vi "BRig_RT_panel_Laser1_v1,10.vi"(7 "input_setValues":bool, 9 "input_dataExp":u16[](array[numeric]), 11 "input_dataLC":u16[](array[numeric])) -> (1 "output_dataExp":u16[](array[numeric]), 3 "output_dataLC":u16[](array[numeric]))   [LabVIEW 2014]
panel:
  in  "Numeric 2":dbl
  in  "Numeric":dbl
  in  "LC_Cue2_PostR_Count":u16
  in  "LC_Cue2_PostR_delayOpt":bool
  in  "LC_Cue2_PostR_Probability":u16
  in  "LC_Cue2_PostR_Block":u16(slide) max=2 step=1 scale=0.0..2.0
  in  "LC_Cue2_PostR_OnOff":bool
  in  "LC_Cue2_PostR_Tdelay":u16
  in  "LC_ENL2_PostR_delayOpt":bool
  in  "LC_ENL2_PostR_Count":u16
  in  "LC_ENL2_PostR_Probability":u16 max=100 step=1
  in  "LC_ENL2_PostR_Block":u16(slide) max=2 step=1 scale=0.0..2.0
  in  "LC_ENL2_PostR_OnOff":bool
  in  "LC_ENL2_PostR_Tdelay":u16
  in  "LC_Cue2_PreR_Count":u16
  in  "LC_Cue2_First_Count":u16
  in  "LC_Cue2_PreR_delayOpt":bool
  in  "LC_ENL2_PreR_delayOpt":bool
  in  "LC_ENL2_PreR_Count":u16
  in  "LC_ENL2_First_Count":u16
  in  "LC_Cue2_First_delayOpt":bool
  in  "LC_ENL2_First_delayOpt":bool
  in  "LC_Cue2_PreR_Probability":u16
  in  "LC_Cue2_PreR_Block":u16(slide) max=2 step=1 scale=0.0..2.0
  in  "LC_Cue2_PreR_OnOff":bool
  in  "LC_Cue2_First_Probability":u16
  in  "LC_Cue2_First_Block":u16(slide) max=2 step=1 scale=0.0..2.0
  in  "LC_Cue2_First_OnOff":bool
  in  "LC_ENL2_PreR_Probability":u16 max=100 step=1
  in  "LC_ENL2_PreR_Block":u16(slide) max=2 step=1 scale=0.0..2.0
  in  "LC_ENL2_PreR_OnOff":bool
  in  "LC_ENL2_First_Probability":u16 max=100 step=1
  in  "LC_ENL2_First_Block":u16(slide) max=2 step=1 scale=0.0..2.0
  in  "LC_Cue2_PreR_Tdelay":u16
  in  "LC_ENL2_PreR_Tdelay":u16
  in  "LC_Cue2_First_Tdelay":u16
  in  "LC_ENL2_First_Tdelay":u16
  in  "LC_ENL2_First_OnOff":bool
  out "LaserPulseTrain":cluster{u16[], u16[]}(graph)
  in  "LED_baseline":bool
  in  "Laser_power_step":dbl
  in  "Laser_power_max":dbl
  in  "Laser_power_min":dbl
  in  "Laser_Tshutter":u16=2
  in  "Laser_Freq":u16=10
  in  "Laser_Tpeak":u16=2
  in  "Laser_T":u16
  in  "LC_Sel_PostR_Count":u16
  in  "LC_Sel_PostR_Probability":u16
  in  "LC_Sel_PostR_Block":u16(slide) max=2 step=1 scale=0.0..2.0
  in  "LC_Sel_PostR_OnOff":bool
  in  "LC_Sel_PostR_Tdelay":u16
  in  "LC_Cue_PostR_Count":u16
  in  "LC_Cue_PostR_delayOpt":bool
  in  "LC_Cue_PostR_Probability":u16
  in  "LC_Cue_PostR_Block":u16(slide) max=2 step=1 scale=0.0..2.0
  in  "LC_Cue_PostR_OnOff":bool
  in  "LC_Cue_PostR_Tdelay":u16
  in  "LC_ENL_PostR_delayOpt":bool
  in  "LC_ENL_PostR_Count":u16
  in  "LC_ENL_PostR_Probability":u16 max=100 step=1
  in  "LC_ENL_PostR_Block":u16(slide) max=2 step=1 scale=0.0..2.0
  in  "LC_ENL_PostR_OnOff":bool
  in  "LC_ENL_PostR_Tdelay":u16
  in  "LC_Sel_PreR_Count":u16
  in  "LC_Sel_First_Count":u16
  in  "LC_Sel_PreR_Probability":u16
  in  "LC_Sel_PreR_Block":u16(slide) max=2 step=1 scale=0.0..2.0
  in  "LC_Sel_PreR_OnOff":bool
  in  "LC_Sel_First_Probability":u16
  in  "LC_Sel_First_Block":u16(slide) max=2 step=1 scale=0.0..2.0
  in  "LC_Sel_First_OnOff":bool
  in  "LC_Sel_PreR_Tdelay":u16
  in  "LC_Sel_First_Tdelay":u16
  in  "LC_Cue_PreR_Count":u16
  in  "LC_Cue_First_Count":u16
  in  "LC_Cue_PreR_delayOpt":bool
  in  "LC_ENL_PreR_delayOpt":bool
  in  "LC_ENL_PreR_Count":u16
  in  "LC_ENL_First_Count":u16
  in  "LC_Cue_First_delayOpt":bool
  in  "LC_ENL_First_delayOpt":bool
  in  "LC_Wrong_Probability":u16
  in  "LC_Wrong_Trial":u16(slide) max=2 step=1 scale=0.0..2.0
  in  "LC_Wrong_Block":u16(slide) max=2 step=1 scale=0.0..2.0
  in  "LC_Wrong_OnOff":bool
  in  "LC_Reward_Probability":u16
  in  "LC_Reward_Trial":u16(slide) max=2 step=1 scale=0.0..2.0
  in  "LC_Reward_Block":u16(slide) max=2 step=1 scale=0.0..2.0
  in  "LC_Reward_OnOff":bool
  in  "LC_Cue_PreR_Probability":u16
  in  "LC_Cue_PreR_Block":u16(slide) max=2 step=1 scale=0.0..2.0
  in  "LC_Cue_PreR_OnOff":bool
  in  "LC_Cue_First_Probability":u16
  in  "LC_Cue_First_Block":u16(slide) max=2 step=1 scale=0.0..2.0
  in  "LC_Cue_First_OnOff":bool
  in  "LC_ENL_PreR_Probability":u16 max=100 step=1
  in  "LC_ENL_PreR_Block":u16(slide) max=2 step=1 scale=0.0..2.0
  in  "LC_ENL_PreR_OnOff":bool
  in  "LC_ENL_First_Probability":u16 max=100 step=1
  in  "LC_ENL_First_Block":u16(slide) max=2 step=1 scale=0.0..2.0
  in  "LC_Wrong_Tdelay":u16
  in  "LC_Cue_PreR_Tdelay":u16
  in  "LC_ENL_PreR_Tdelay":u16
  in  "LC_Reward_Tdelay":u16
  in  "LC_Cue_First_Tdelay":u16
  in  "LC_ENL_First_Tdelay":u16
  in  "LC_ENL_First_OnOff":bool
  # "Laser1 Control\n                               On/Off      Block        Probability [%]   Delay [ms]                              Count"
  # "On/Off      Block        Probability [%]   Delay [ms]                              Count"
  # "Enforced\nNonLick"
  # "Enforced\nNonLick\n     2"
  # "from end"
  # "from end"
  # "First\nTrial"
  # "First\nTrial"
  # "from start"
  # "from start"
  # "from end"
  # "from end"
  # "PreReward\nTrials"
  # "PreReward\nTrials"
  # "from start"
  # "from start"
  # "from end"
  # "from end"
  # "PostReward\nTrials"
  # "PostReward\nTrials"
  # "from start"
  # "from start"
  # "Cue"
  # "Cue\n  2"
  # "from end"
  # "from end"
  # "First\nTrial"
  # "First\nTrial"
  # "from start"
  # "from start"
  # "from end"
  # "from end"
  # "PreReward\nTrials"
  # "PreReward\nTrials"
  # "from start"
  # "from start"
  # "from end"
  # "from end"
  # "PostReward\nTrials"
  # "PostReward\nTrials"
  # "from start"
  # "from start"
  # "Selection"
  # "from start"
  # "First\nTrial"
  # "from start"
  # "PreReward\nTrials"
  # "from start"
  # "PostReward\nTrials"
  # "Laser1 Parameters"
  # "Laser1 Response\n           On/Off      Block           Trial     Probability %  Delay [ms]"
  # "Frequency\n[Hz]"
  # "Selection\nReward"
  # "Timing [ms]\n Duration     Peak Width   Shutter"
  # "Selection\nWrong"
  # "Laser Power [V]\nMin          Max              Step"
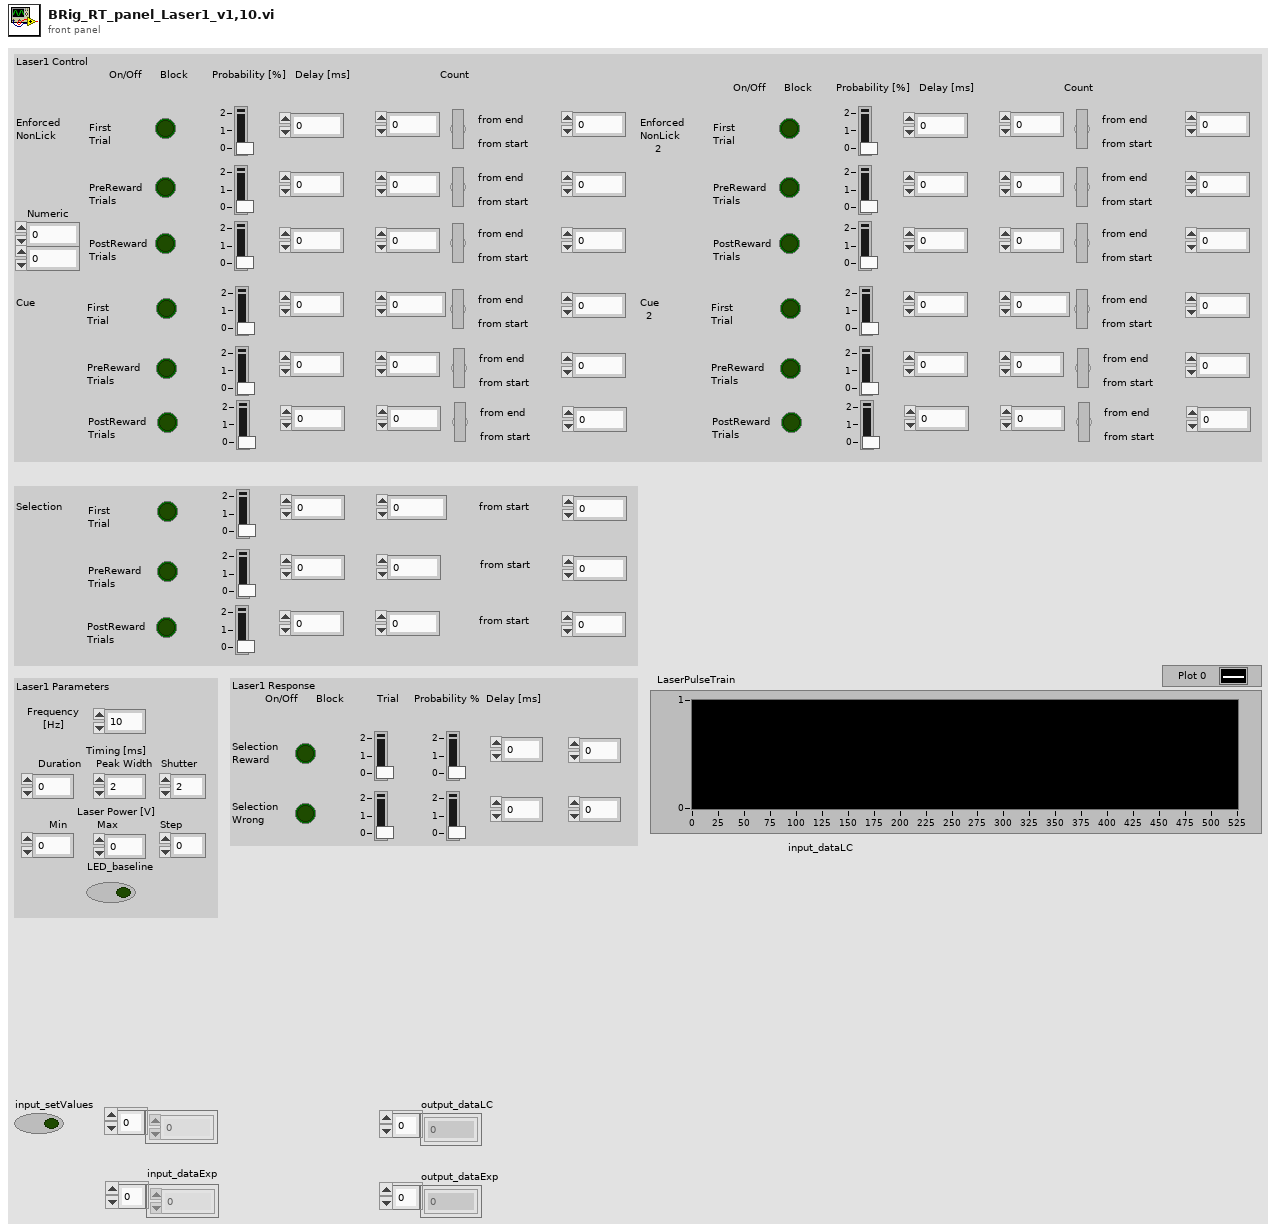
[diagram p1: front panel]
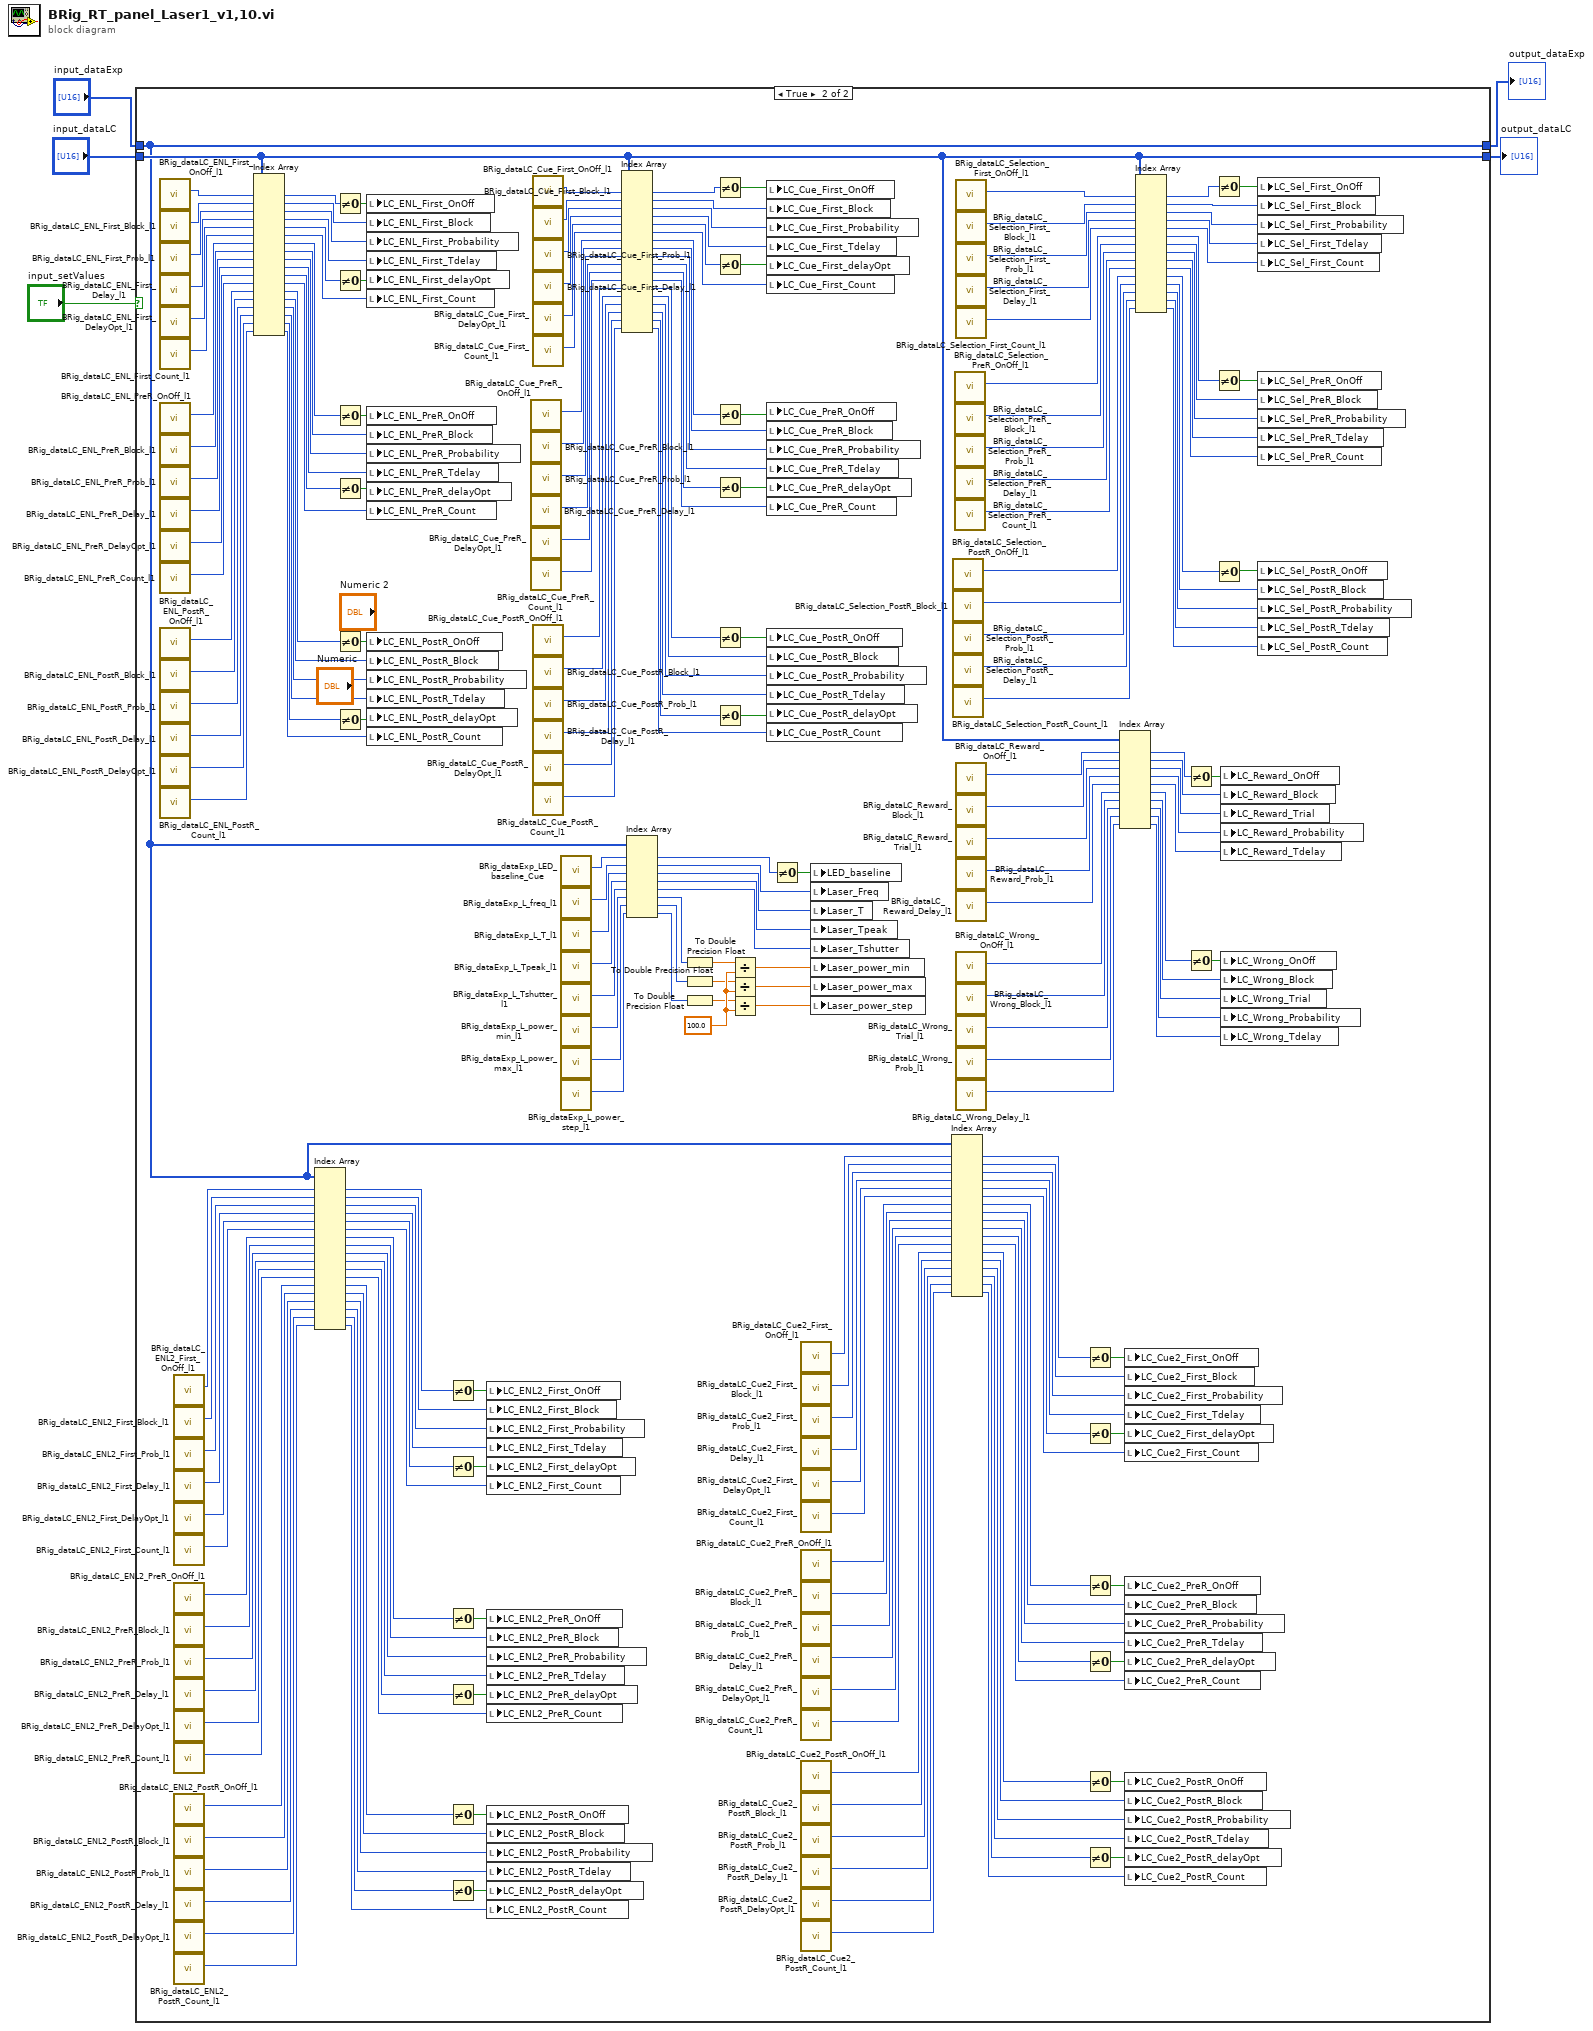
[diagram p0: block diagram]
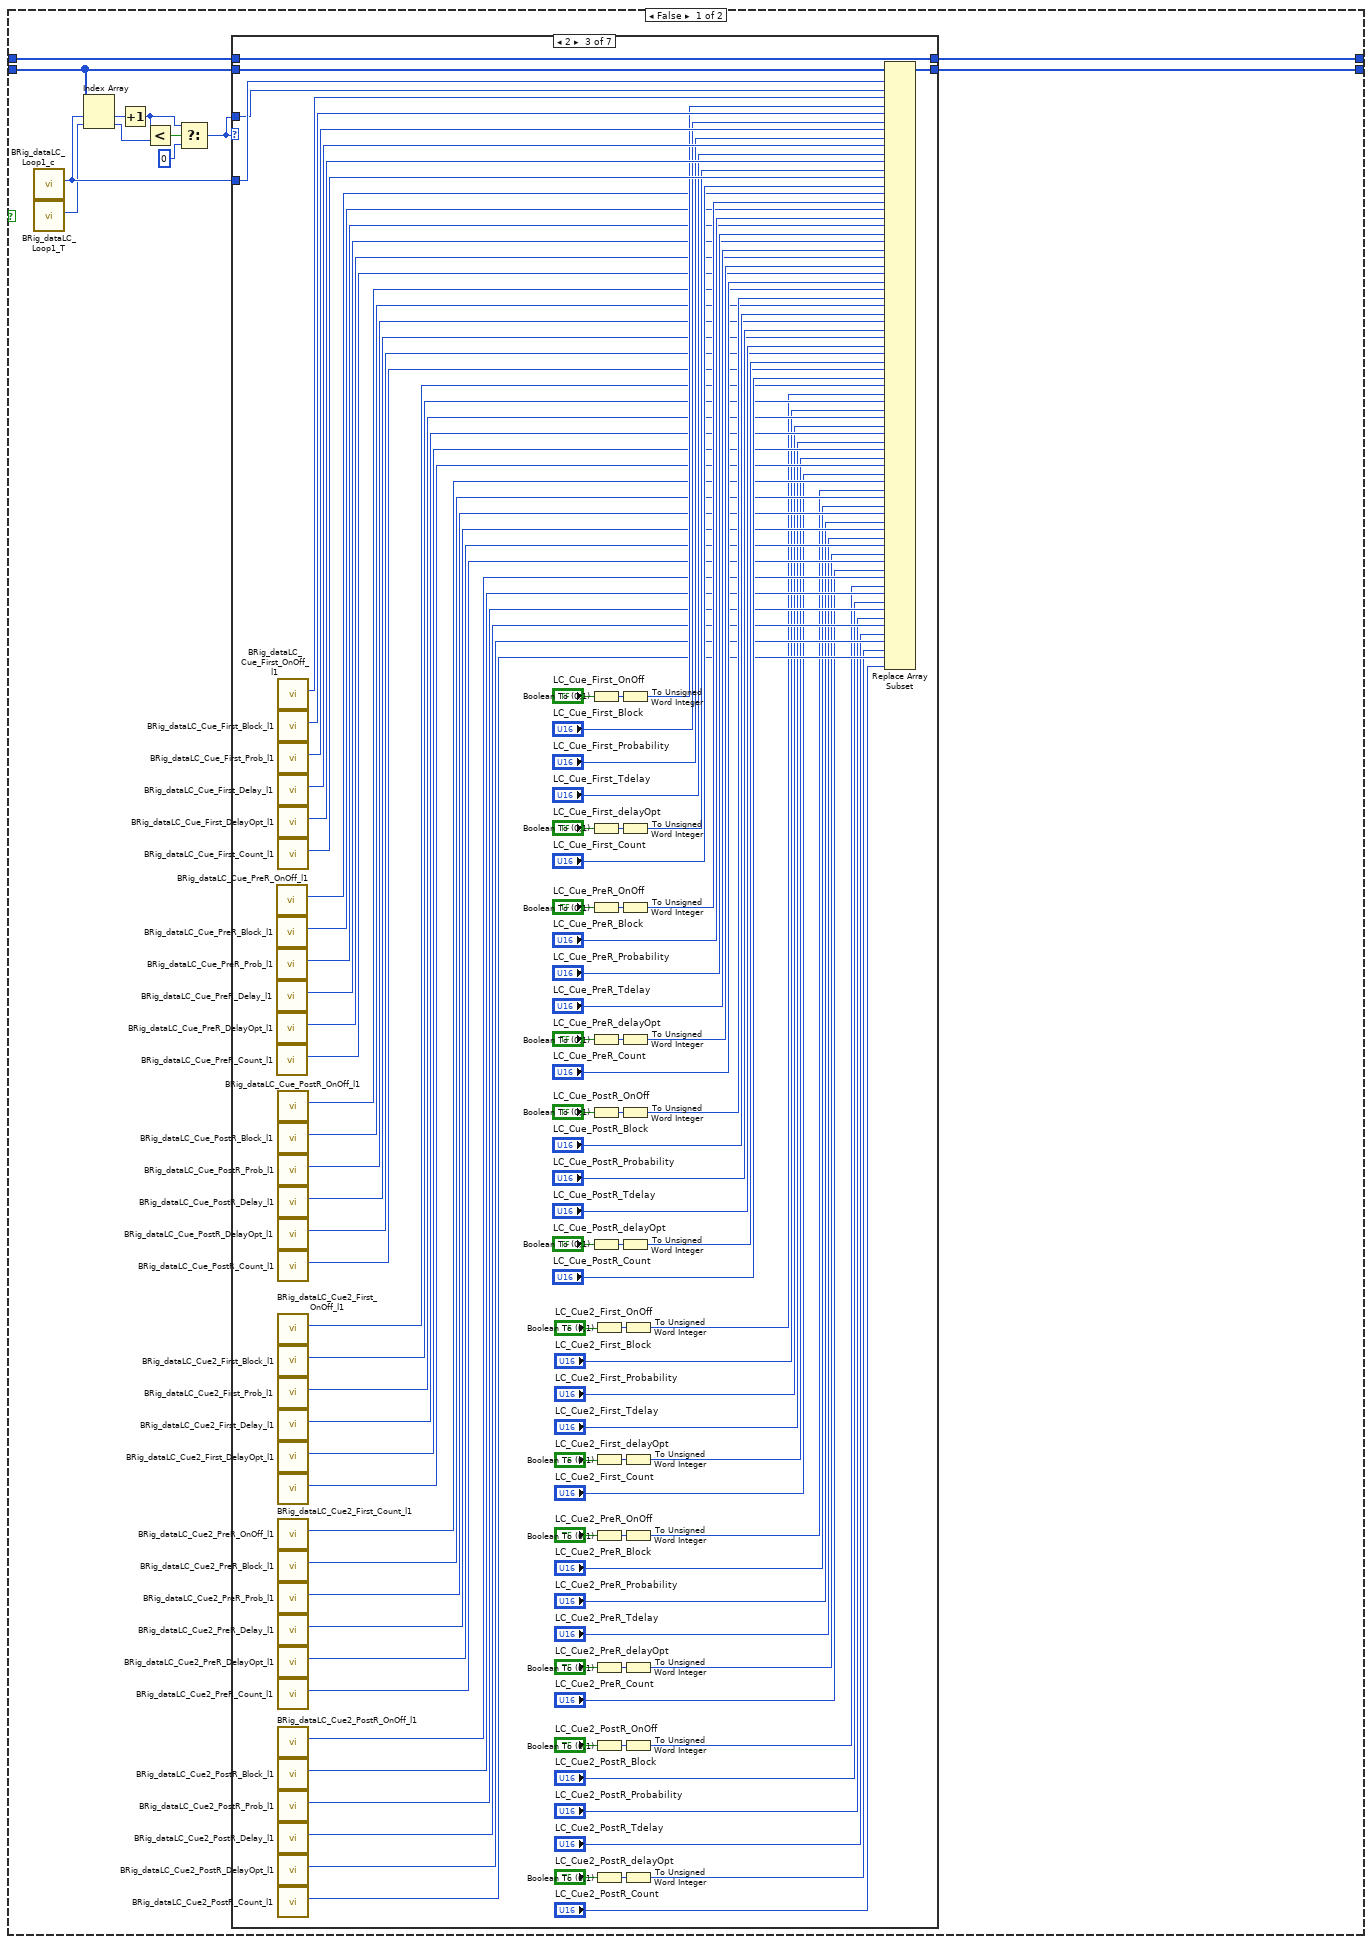
[diagram p2: hidden frame]
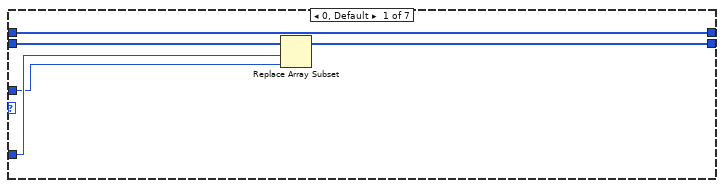
[diagram p3: hidden frame]
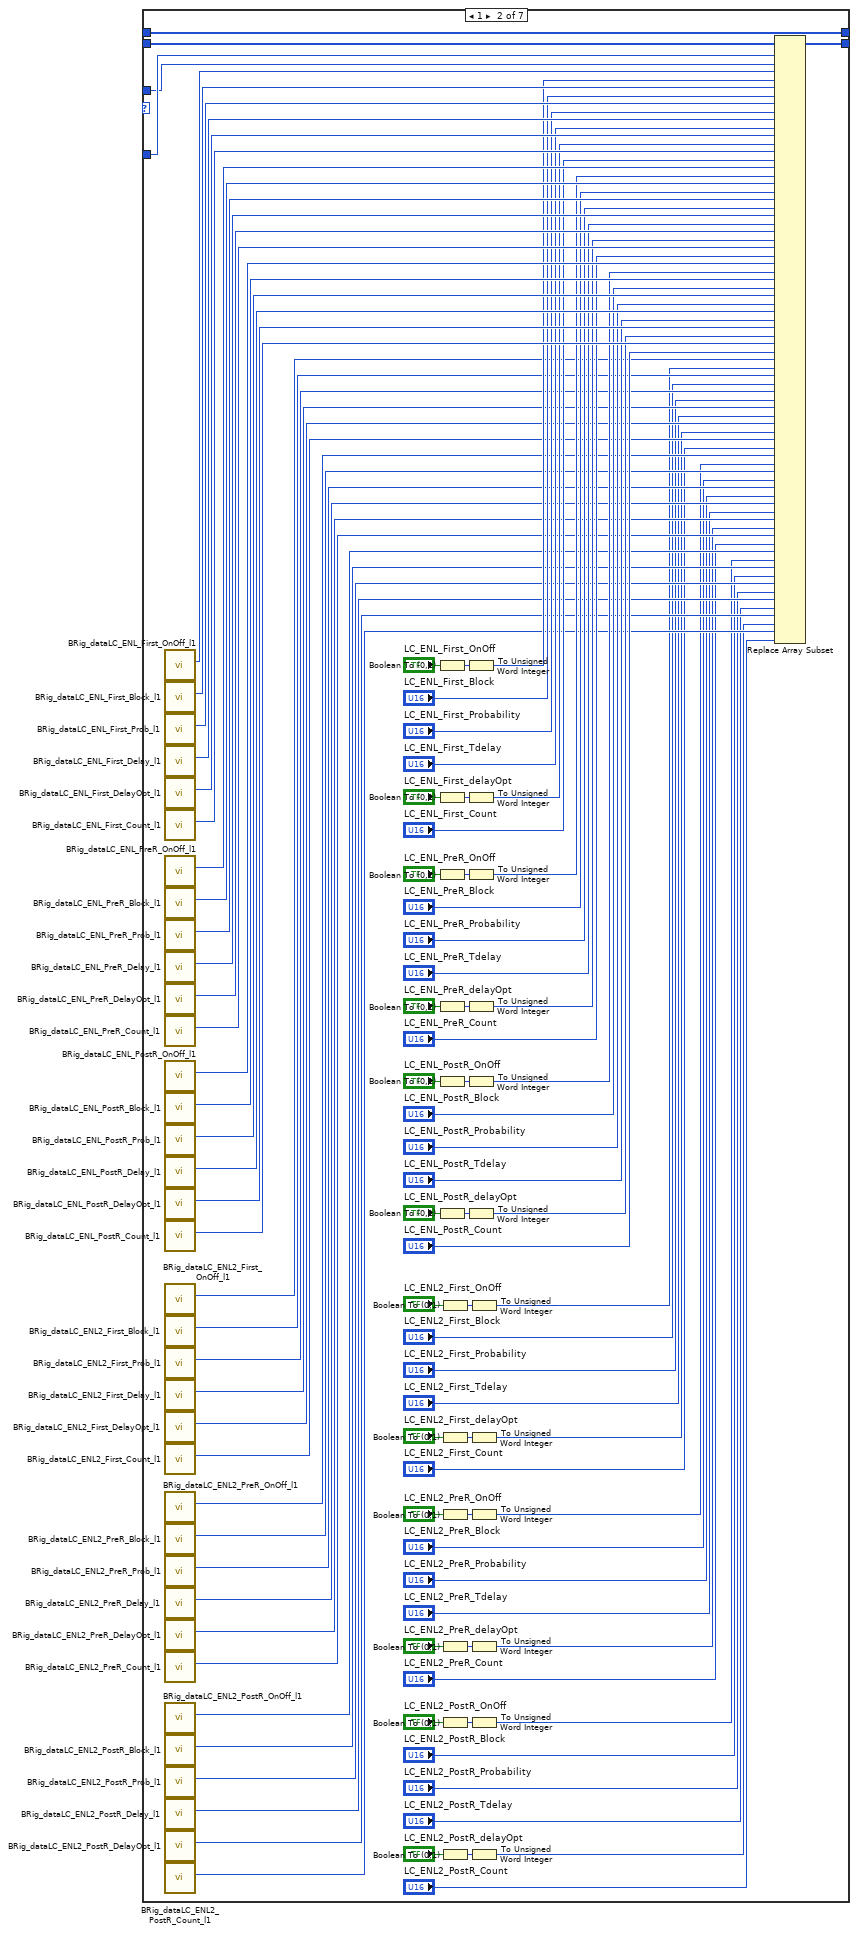
[diagram p4: hidden frame]
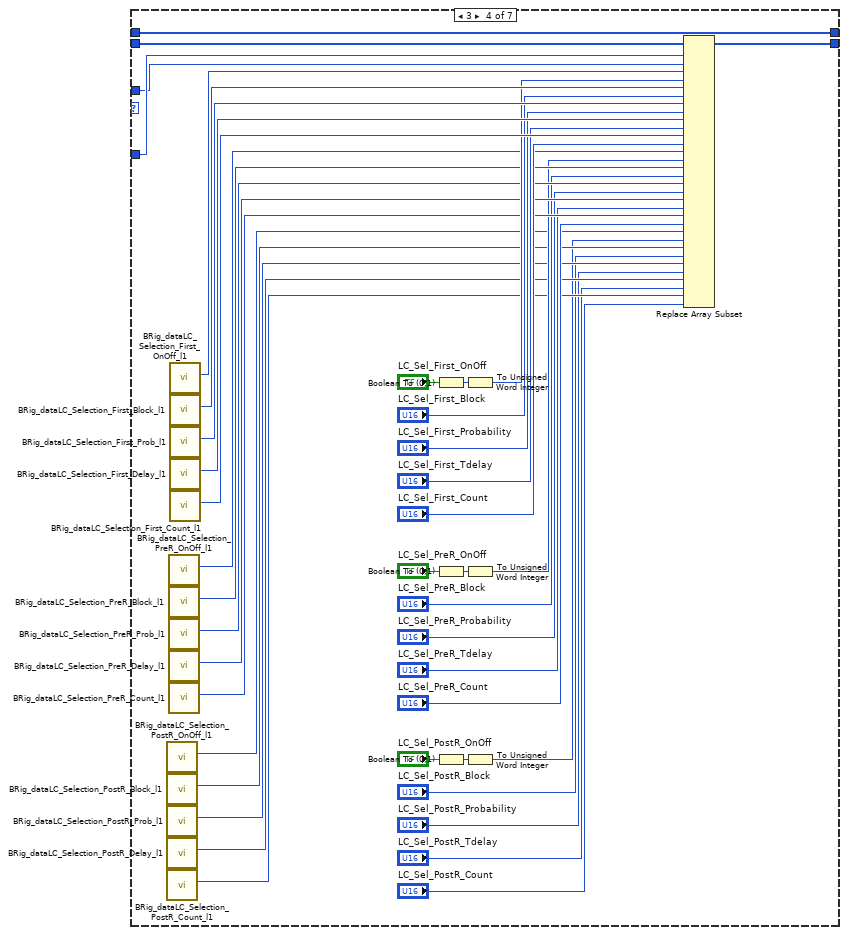
[diagram p5: hidden frame]
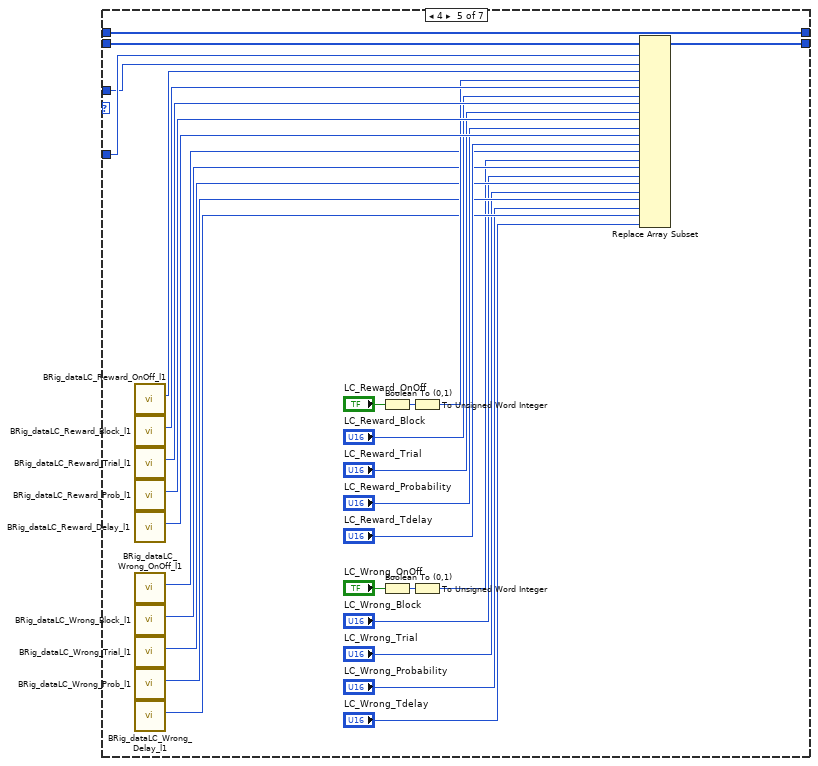
[diagram p6: hidden frame]
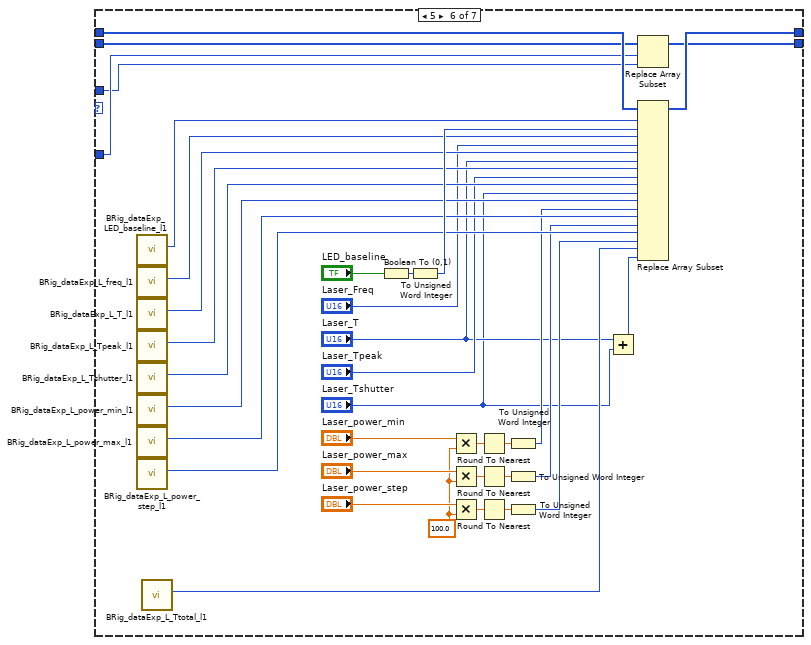
[diagram p7: hidden frame]
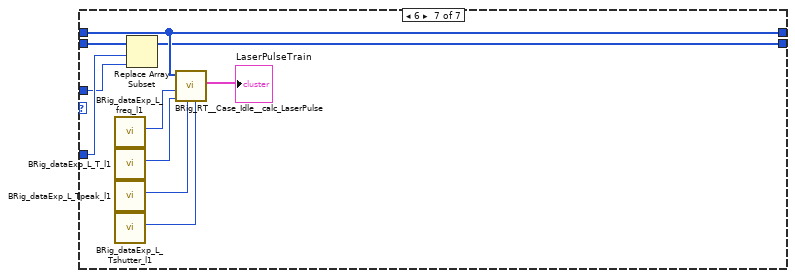
[diagram p8: hidden frame]
diagram:
  n1 = case shown="True" "input_setValues" {
    tunnel: "input_dataLC" -> [w17 w462]
    tunnel: [w11 w462] -> w4
    tunnel: "input_dataExp" -> [w7 w377]
    tunnel: [w6 w377] -> w1
    frame False {
      n2 = call "BRig_dataLC_Loop1_c.vi"() -> ("output_Loop1_c"=w10:i32)  [unwired: 11 in]
      n3 = call "BRig_dataLC_Loop1_T.vi"() -> ("output_Loop1_T"=w9:i32)  [unwired: 11 in]
      n4 = Index Array(array=w17, index #1=w10, index #2=w9) -> (element #1=w16:u16, element #2=w15:u16)
      n5 = Increment(x=w16) -> (x+1=w12:u16)
      n6 = Less?(x=w12, y=w15) -> (x < y?=w14:bool)
      n7 = Select(t=w12, s=w14, f=u16 0) -> (s? t:f=w8:u16)
      n8 = case shown="2" w8 {
        tunnel: w17 -> [w22 w123 w224 w265 w294 w299 w338]
        tunnel: w10 -> [w20 w73 w186 w227 w268 w297 w336]
        tunnel: w8 -> [w19 w72 w185 w226 w267 w296 w335]
        tunnel: [w21 w116 w223 w264 w293 w298 w337] -> w11
        tunnel: w7 -> [w18 w71 w172 w225 w266 w301 w340]
        tunnel: [w18 w71 w172 w225 w266 w300 w340] -> w6
        frame 0, Default {
          n9 = Replace Array Subset(array=w22, new element=w19, index=w20) -> (w21:u16[])
        }
        frame 1 {
          n10 = call "BRig_dataLC_ENL_First_OnOff_l1.vi"() -> ("output_ENL_First_OnOff"=w122:i32)  [unwired: 11 in]
          n11 = call "BRig_dataLC_ENL_First_Block_l1.vi"() -> ("output_ENL_First_Block"=w121:i32)  [unwired: 11 in]
          n12 = call "BRig_dataLC_ENL_First_Prob_l1.vi"() -> ("output_ENL_First_Prob"=w120:i32)  [unwired: 11 in]
          n13 = call "BRig_dataLC_ENL_First_Delay_l1.vi"() -> ("output_ENL_First_Delay"=w119:i32)  [unwired: 11 in]
          n14 = call "BRig_dataLC_ENL_First_DelayOpt_l1.vi"() -> ("output_ENL_First_DelayOpt"=w118:i32)  [unwired: 11 in]
          n15 = call "BRig_dataLC_ENL_First_Count_l1.vi"() -> ("output_ENL_First_Count"=w117:i32)  [unwired: 11 in]
          n16 = call "BRig_dataLC_ENL_PreR_OnOff_l1.vi"() -> ("output_ENL_PreR_OnOff"=w115:i32)  [unwired: 11 in]
          n17 = call "BRig_dataLC_ENL_PreR_Block_l1.vi"() -> ("output_ENL_PreR_Block"=w114:i32)  [unwired: 11 in]
          n18 = call "BRig_dataLC_ENL_PreR_Prob_l1.vi"() -> ("output_ENL_PreR_Prob"=w113:i32)  [unwired: 11 in]
          n19 = call "BRig_dataLC_ENL_PreR_Delay_l1.vi"() -> ("output_ENL_PreR_Delay"=w112:i32)  [unwired: 11 in]
          n20 = call "BRig_dataLC_ENL_PreR_DelayOpt_l1.vi"() -> ("output_ENL_PreR_DelayOpt"=w111:i32)  [unwired: 11 in]
          n21 = call "BRig_dataLC_ENL_PreR_Count_l1.vi"() -> ("output_ENL_PreR_Count"=w110:i32)  [unwired: 11 in]
          n22 = call "BRig_dataLC_ENL_PostR_OnOff_l1.vi"() -> ("output_ENL_PostR_OnOff"=w109:i32)  [unwired: 11 in]
          n23 = call "BRig_dataLC_ENL_PostR_Block_l1.vi"() -> ("output_ENL_PostR_Block"=w108:i32)  [unwired: 11 in]
          n24 = call "BRig_dataLC_ENL_PostR_Prob_l1.vi"() -> ("output_ENL_PostR_Prob"=w107:i32)  [unwired: 11 in]
          n25 = call "BRig_dataLC_ENL_PostR_Delay_l1.vi"() -> ("output_ENL_PostR_Delay"=w106:i32)  [unwired: 11 in]
          n26 = call "BRig_dataLC_ENL_PostR_DelayOpt_l1.vi"() -> ("output_ENL_PostR_DelayOpt"=w105:i32)  [unwired: 11 in]
          n27 = call "BRig_dataLC_ENL_PostR_Count_l1.vi"() -> ("output_ENL_PostR_Count"=w104:i32)  [unwired: 11 in]
          n28 = call "BRig_dataLC_ENL2_First_OnOff_l1.vi"() -> ("output_ENL2_First_OnOff"=w70:i32)  [unwired: 11 in]
          n29 = call "BRig_dataLC_ENL2_First_Block_l1.vi"() -> ("output_ENL2_First_Block"=w69:i32)  [unwired: 11 in]
          n30 = call "BRig_dataLC_ENL2_First_Prob_l1.vi"() -> ("output_ENL2_First_Prob"=w68:i32)  [unwired: 11 in]
          n31 = call "BRig_dataLC_ENL2_First_Delay_l1.vi"() -> ("output_ENL2_First_Delay"=w67:i32)  [unwired: 11 in]
          n32 = call "BRig_dataLC_ENL2_First_DelayOpt_l1.vi"() -> ("output_ENL2_First_DelayOpt"=w66:i32)  [unwired: 11 in]
          n33 = call "BRig_dataLC_ENL2_First_Count_l1.vi"() -> ("output_ENL2_First_Count"=w65:i32)  [unwired: 11 in]
          n34 = call "BRig_dataLC_ENL2_PreR_OnOff_l1.vi"() -> ("output_ENL2_PreR_OnOff"=w64:i32)  [unwired: 11 in]
          n35 = call "BRig_dataLC_ENL2_PreR_Block_l1.vi"() -> ("output_ENL2_PreR_Block"=w63:i32)  [unwired: 11 in]
          n36 = call "BRig_dataLC_ENL2_PreR_Prob_l1.vi"() -> ("output_ENL2_PreR_Prob"=w62:i32)  [unwired: 11 in]
          n37 = call "BRig_dataLC_ENL2_PreR_Delay_l1.vi"() -> ("output_ENL2_PreR_Delay"=w61:i32)  [unwired: 11 in]
          n38 = call "BRig_dataLC_ENL2_PreR_DelayOpt_l1.vi"() -> ("output_ENL2_PreR_DelayOpt"=w60:i32)  [unwired: 11 in]
          n39 = call "BRig_dataLC_ENL2_PreR_Count_l1.vi"() -> ("output_ENL2_PreR_Count"=w59:i32)  [unwired: 11 in]
          n40 = call "BRig_dataLC_ENL2_PostR_OnOff_l1.vi"() -> ("output_ENL2_PostR_OnOff"=w58:i32)  [unwired: 11 in]
          n41 = call "BRig_dataLC_ENL2_PostR_Block_l1.vi"() -> ("output_ENL2_PostR_Block"=w57:i32)  [unwired: 11 in]
          n42 = call "BRig_dataLC_ENL2_PostR_Prob_l1.vi"() -> ("output_ENL2_PostR_Prob"=w56:i32)  [unwired: 11 in]
          n43 = call "BRig_dataLC_ENL2_PostR_Delay_l1.vi"() -> ("output_ENL2_PostR_Delay"=w55:i32)  [unwired: 11 in]
          n44 = call "BRig_dataLC_ENL2_PostR_DelayOpt_l1.vi"() -> ("output_ENL2_PostR_DelayOpt"=w54:i32)  [unwired: 11 in]
          n45 = call "BRig_dataLC_ENL2_PostR_Count_l1.vi"() -> ("output_ENL2_PostR_Count"=w53:i32)  [unwired: 11 in]
          n46 = Boolean To (0,1)(Boolean="LC_ENL_First_OnOff") -> (0, 1=w102:i16)
          n47 = Boolean To (0,1)(Boolean="LC_ENL_First_delayOpt") -> (0, 1=w101:i16)
          n48 = Boolean To (0,1)(Boolean="LC_ENL_PreR_OnOff") -> (0, 1=w99:i16)
          n49 = Boolean To (0,1)(Boolean="LC_ENL_PreR_delayOpt") -> (0, 1=w97:i16)
          n50 = Boolean To (0,1)(Boolean="LC_ENL_PostR_OnOff") -> (0, 1=w95:i16)
          n51 = Boolean To (0,1)(Boolean="LC_ENL_PostR_delayOpt") -> (0, 1=w93:i16)
          n52 = Boolean To (0,1)(Boolean="LC_ENL2_First_OnOff") -> (0, 1=w43:i16)
          n53 = Boolean To (0,1)(Boolean="LC_ENL2_First_delayOpt") -> (0, 1=w42:i16)
          n54 = Boolean To (0,1)(Boolean="LC_ENL2_PreR_OnOff") -> (0, 1=w41:i16)
          n55 = Boolean To (0,1)(Boolean="LC_ENL2_PreR_delayOpt") -> (0, 1=w39:i16)
          n56 = Boolean To (0,1)(Boolean="LC_ENL2_PostR_OnOff") -> (0, 1=w31:i16)
          n57 = Boolean To (0,1)(Boolean="LC_ENL2_PostR_delayOpt") -> (0, 1=w29:i16)
          n58 = To Unsigned Word Integer(number=w102) -> (unsigned 16bit integer=w91:u16)
          n59 = To Unsigned Word Integer(number=w101) -> (unsigned 16bit integer=w87:u16)
          n60 = To Unsigned Word Integer(number=w99) -> (unsigned 16bit integer=w85:u16)
          n61 = To Unsigned Word Integer(number=w97) -> (unsigned 16bit integer=w81:u16)
          n62 = To Unsigned Word Integer(number=w95) -> (unsigned 16bit integer=w79:u16)
          n63 = To Unsigned Word Integer(number=w93) -> (unsigned 16bit integer=w75:u16)
          n64 = To Unsigned Word Integer(number=w43) -> (unsigned 16bit integer=w50:u16)
          n65 = To Unsigned Word Integer(number=w42) -> (unsigned 16bit integer=w46:u16)
          n66 = To Unsigned Word Integer(number=w41) -> (unsigned 16bit integer=w44:u16)
          n67 = To Unsigned Word Integer(number=w39) -> (unsigned 16bit integer=w34:u16)
          n68 = To Unsigned Word Integer(number=w31) -> (unsigned 16bit integer=w32:u16)
          n69 = To Unsigned Word Integer(number=w29) -> (unsigned 16bit integer=w24:u16)
          n70 = Replace Array Subset(array=w123, new element #1=w72, index #1=w73, new element #2=w91, index #2=w122, new element #3="LC_ENL_First_Block", index #3=w121, new element #4="LC_ENL_First_Probability", index #4=w120, new element #5="LC_ENL_First_Tdelay", index #5=w119, new element #6=w87, index #6=w118, new element #7="LC_ENL_First_Count", index #7=w117, new element #8=w85, index #8=w115, new element #9="LC_ENL_PreR_Block", index #9=w114, new element #10="LC_ENL_PreR_Probability", index #10=w113, new element #11="LC_ENL_PreR_Tdelay", index #11=w112, new element #12=w81, index #12=w111, new element #13="LC_ENL_PreR_Count", index #13=w110, new element #14=w79, index #14=w109, new element #15="LC_ENL_PostR_Block", index #15=w108, new element #16="LC_ENL_PostR_Probability", index #16=w107, new element #17="LC_ENL_PostR_Tdelay", index #17=w106, new element #18=w75, index #18=w105, new element #19="LC_ENL_PostR_Count", index #19=w104, new element #20=w50, index #20=w70, new element #21="LC_ENL2_First_Block", index #21=w69, new element #22="LC_ENL2_First_Probability", index #22=w68, new element #23="LC_ENL2_First_Tdelay", index #23=w67, new element #24=w46, index #24=w66, new element #25="LC_ENL2_First_Count", index #25=w65, new element #26=w44, index #26=w64, new element #27="LC_ENL2_PreR_Block", index #27=w63, new element #28="LC_ENL2_PreR_Probability", index #28=w62, new element #29="LC_ENL2_PreR_Tdelay", index #29=w61, new element #30=w34, index #30=w60, new element #31="LC_ENL2_PreR_Count", index #31=w59, new element #32=w32, index #32=w58, new element #33="LC_ENL2_PostR_Block", index #33=w57, new element #34="LC_ENL2_PostR_Probability", index #34=w56, new element #35="LC_ENL2_PostR_Tdelay", index #35=w55, new element #36=w24, index #36=w54, new element #37="LC_ENL2_PostR_Count", index #37=w53) -> (w116:u16[])
        }
        frame 2 {
          n71 = call "BRig_dataLC_Cue_PreR_OnOff_l1.vi"() -> ("output_Cue_PreR_OnOff"=w182:i32)  [unwired: 11 in]
          n72 = call "BRig_dataLC_Cue_PreR_Block_l1.vi"() -> ("output_Cue_PreR_Block"=w181:i32)  [unwired: 11 in]
          n73 = call "BRig_dataLC_Cue_PreR_Prob_l1.vi"() -> ("output_Cue_PreR_Prob"=w180:i32)  [unwired: 11 in]
          n74 = call "BRig_dataLC_Cue_PreR_Delay_l1.vi"() -> ("output_Cue_PreR_Delay"=w179:i32)  [unwired: 11 in]
          n75 = call "BRig_dataLC_Cue_PreR_DelayOpt_l1.vi"() -> ("output_Cue_PreR_DelayOpt"=w178:i32)  [unwired: 11 in]
          n76 = call "BRig_dataLC_Cue_PreR_Count_l1.vi"() -> ("output_Cue_PreR_Count"=w183:i32)  [unwired: 11 in]
          n77 = call "BRig_dataLC_Cue_First_OnOff_l1.vi"() -> ("output_Cue_First_OnOff"=w222:i32)  [unwired: 11 in]
          n78 = call "BRig_dataLC_Cue_First_Block_l1.vi"() -> ("output_Cue_First_Block"=w221:i32)  [unwired: 11 in]
          n79 = call "BRig_dataLC_Cue_First_Prob_l1.vi"() -> ("output_Cue_First_Prob"=w220:i32)  [unwired: 11 in]
          n80 = call "BRig_dataLC_Cue_First_Delay_l1.vi"() -> ("output_Cue_First_Delay"=w219:i32)  [unwired: 11 in]
          n81 = call "BRig_dataLC_Cue_First_DelayOpt_l1.vi"() -> ("output_Cue_First_DelayOpt"=w218:i32)  [unwired: 11 in]
          n82 = call "BRig_dataLC_Cue_First_Count_l1.vi"() -> ("output_Cue_First_Count"=w217:i32)  [unwired: 11 in]
          n83 = call "BRig_dataLC_Cue_PostR_OnOff_l1.vi"() -> ("output_Cue_PostR_OnOff"=w184:i32)  [unwired: 11 in]
          n84 = call "BRig_dataLC_Cue_PostR_Block_l1.vi"() -> ("output_Cue_PostR_Block"=w177:i32)  [unwired: 11 in]
          n85 = call "BRig_dataLC_Cue_PostR_Prob_l1.vi"() -> ("output_Cue_PostR_Prob"=w176:i32)  [unwired: 11 in]
          n86 = call "BRig_dataLC_Cue_PostR_Delay_l1.vi"() -> ("output_Cue_PostR_Delay"=w175:i32)  [unwired: 11 in]
          n87 = call "BRig_dataLC_Cue_PostR_DelayOpt_l1.vi"() -> ("output_Cue_PostR_DelayOpt"=w174:i32)  [unwired: 11 in]
          n88 = call "BRig_dataLC_Cue_PostR_Count_l1.vi"() -> ("output_Cue_PostR_Count"=w173:i32)  [unwired: 11 in]
          n89 = call "BRig_dataLC_Cue2_First_OnOff_l1.vi"() -> ("output_Cue2_First_OnOff"=w171:i32)  [unwired: 11 in]
          n90 = call "BRig_dataLC_Cue2_First_Block_l1.vi"() -> ("output_Cue2_First_Block"=w170:i32)  [unwired: 11 in]
          n91 = call "BRig_dataLC_Cue2_First_Prob_l1.vi"() -> ("output_Cue2_First_Prob"=w169:i32)  [unwired: 11 in]
          n92 = call "BRig_dataLC_Cue2_First_Delay_l1.vi"() -> ("output_Cue2_First_Delay"=w168:i32)  [unwired: 11 in]
          n93 = call "BRig_dataLC_Cue2_First_DelayOpt_l1.vi"() -> ("output_Cue2_First_DelayOpt"=w167:i32)  [unwired: 11 in]
          n94 = call "BRig_dataLC_Cue2_First_Count_l1.vi"() -> ("output_Cue2_First_Count"=w166:i32)  [unwired: 11 in]
          n95 = call "BRig_dataLC_Cue2_PreR_OnOff_l1.vi"() -> ("output_Cue2_PreR_OnOff"=w165:i32)  [unwired: 11 in]
          n96 = call "BRig_dataLC_Cue2_PreR_Block_l1.vi"() -> ("output_Cue2_PreR_Block"=w164:i32)  [unwired: 11 in]
          n97 = call "BRig_dataLC_Cue2_PreR_Prob_l1.vi"() -> ("output_Cue2_PreR_Prob"=w163:i32)  [unwired: 11 in]
          n98 = call "BRig_dataLC_Cue2_PreR_Delay_l1.vi"() -> ("output_Cue2_PreR_Delay"=w162:i32)  [unwired: 11 in]
          n99 = call "BRig_dataLC_Cue2_PreR_DelayOpt_l1.vi"() -> ("output_Cue2_PreR_DelayOpt"=w161:i32)  [unwired: 11 in]
          n100 = call "BRig_dataLC_Cue2_PreR_Count_l1.vi"() -> ("output_Cue2_PreR_Count"=w160:i32)  [unwired: 11 in]
          n101 = call "BRig_dataLC_Cue2_PostR_OnOff_l1.vi"() -> ("output_Cue2_PostR_OnOff"=w159:i32)  [unwired: 11 in]
          n102 = call "BRig_dataLC_Cue2_PostR_Block_l1.vi"() -> ("output_Cue2_PostR_Block"=w158:i32)  [unwired: 11 in]
          n103 = call "BRig_dataLC_Cue2_PostR_Prob_l1.vi"() -> ("output_Cue2_PostR_Prob"=w157:i32)  [unwired: 11 in]
          n104 = call "BRig_dataLC_Cue2_PostR_Delay_l1.vi"() -> ("output_Cue2_PostR_Delay"=w156:i32)  [unwired: 11 in]
          n105 = call "BRig_dataLC_Cue2_PostR_DelayOpt_l1.vi"() -> ("output_Cue2_PostR_DelayOpt"=w155:i32)  [unwired: 11 in]
          n106 = call "BRig_dataLC_Cue2_PostR_Count_l1.vi"() -> ("output_Cue2_PostR_Count"=w154:i32)  [unwired: 11 in]
          n107 = Boolean To (0,1)(Boolean="LC_Cue_First_OnOff") -> (0, 1=w210:i16)
          n108 = Boolean To (0,1)(Boolean="LC_Cue_First_delayOpt") -> (0, 1=w209:i16)
          n109 = Boolean To (0,1)(Boolean="LC_Cue_PreR_OnOff") -> (0, 1=w208:i16)
          n110 = Boolean To (0,1)(Boolean="LC_Cue_PreR_delayOpt") -> (0, 1=w207:i16)
          n111 = Boolean To (0,1)(Boolean="LC_Cue_PostR_OnOff") -> (0, 1=w206:i16)
          n112 = Boolean To (0,1)(Boolean="LC_Cue_PostR_delayOpt") -> (0, 1=w205:i16)
          n113 = Boolean To (0,1)(Boolean="LC_Cue2_First_OnOff") -> (0, 1=w153:i16)
          n114 = Boolean To (0,1)(Boolean="LC_Cue2_First_delayOpt") -> (0, 1=w152:i16)
          n115 = Boolean To (0,1)(Boolean="LC_Cue2_PreR_OnOff") -> (0, 1=w151:i16)
          n116 = Boolean To (0,1)(Boolean="LC_Cue2_PreR_delayOpt") -> (0, 1=w150:i16)
          n117 = Boolean To (0,1)(Boolean="LC_Cue2_PostR_OnOff") -> (0, 1=w149:i16)
          n118 = Boolean To (0,1)(Boolean="LC_Cue2_PostR_delayOpt") -> (0, 1=w148:i16)
          n119 = To Unsigned Word Integer(number=w210) -> (unsigned 16bit integer=w204:u16)
          n120 = To Unsigned Word Integer(number=w209) -> (unsigned 16bit integer=w200:u16)
          n121 = To Unsigned Word Integer(number=w208) -> (unsigned 16bit integer=w198:u16)
          n122 = To Unsigned Word Integer(number=w207) -> (unsigned 16bit integer=w194:u16)
          n123 = To Unsigned Word Integer(number=w206) -> (unsigned 16bit integer=w192:u16)
          n124 = To Unsigned Word Integer(number=w205) -> (unsigned 16bit integer=w188:u16)
          n125 = To Unsigned Word Integer(number=w153) -> (unsigned 16bit integer=w141:u16)
          n126 = To Unsigned Word Integer(number=w152) -> (unsigned 16bit integer=w137:u16)
          n127 = To Unsigned Word Integer(number=w151) -> (unsigned 16bit integer=w135:u16)
          n128 = To Unsigned Word Integer(number=w150) -> (unsigned 16bit integer=w131:u16)
          n129 = To Unsigned Word Integer(number=w149) -> (unsigned 16bit integer=w129:u16)
          n130 = To Unsigned Word Integer(number=w148) -> (unsigned 16bit integer=w125:u16)
          n131 = Replace Array Subset(array=w224, new element #1=w185, index #1=w186, new element #2=w204, index #2=w222, new element #3="LC_Cue_First_Block", index #3=w221, new element #4="LC_Cue_First_Probability", index #4=w220, new element #5="LC_Cue_First_Tdelay", index #5=w219, new element #6=w200, index #6=w218, new element #7="LC_Cue_First_Count", index #7=w217, new element #8=w198, index #8=w182, new element #9="LC_Cue_PreR_Block", index #9=w181, new element #10="LC_Cue_PreR_Probability", index #10=w180, new element #11="LC_Cue_PreR_Tdelay", index #11=w179, new element #12=w194, index #12=w178, new element #13="LC_Cue_PreR_Count", index #13=w183, new element #14=w192, index #14=w184, new element #15="LC_Cue_PostR_Block", index #15=w177, new element #16="LC_Cue_PostR_Probability", index #16=w176, new element #17="LC_Cue_PostR_Tdelay", index #17=w175, new element #18=w188, index #18=w174, new element #19="LC_Cue_PostR_Count", index #19=w173, new element #20=w141, index #20=w171, new element #21="LC_Cue2_First_Block", index #21=w170, new element #22="LC_Cue2_First_Probability", index #22=w169, new element #23="LC_Cue2_First_Tdelay", index #23=w168, new element #24=w137, index #24=w167, new element #25="LC_Cue2_First_Count", index #25=w166, new element #26=w135, index #26=w165, new element #27="LC_Cue2_PreR_Block", index #27=w164, new element #28="LC_Cue2_PreR_Probability", index #28=w163, new element #29="LC_Cue2_PreR_Tdelay", index #29=w162, new element #30=w131, index #30=w161, new element #31="LC_Cue2_PreR_Count", index #31=w160, new element #32=w129, index #32=w159, new element #33="LC_Cue2_PostR_Block", index #33=w158, new element #34="LC_Cue2_PostR_Probability", index #34=w157, new element #35="LC_Cue2_PostR_Tdelay", index #35=w156, new element #36=w125, index #36=w155, new element #37="LC_Cue2_PostR_Count", index #37=w154) -> (w223:u16[])
        }
        frame 3 {
          n132 = call "BRig_dataLC_Selection_PostR_OnOff_l1.vi"() -> ("output_Selection_PostR_OnOff"=w237:i32)  [unwired: 11 in]
          n133 = call "BRig_dataLC_Selection_PostR_Block_l1.vi"() -> ("output_Selection_PostR_Block"=w236:i32)  [unwired: 11 in]
          n134 = call "BRig_dataLC_Selection_PostR_Prob_l1.vi"() -> ("output_Selection_PostR_Prob"=w235:i32)  [unwired: 11 in]
          n135 = call "BRig_dataLC_Selection_PostR_Delay_l1.vi"() -> ("output_Selection_PostR_Delay"=w234:i32)  [unwired: 11 in]
          n136 = call "BRig_dataLC_Selection_PostR_Count_l1.vi"() -> ("output_Selection_PostR_Count"=w233:i32)  [unwired: 11 in]
          n137 = call "BRig_dataLC_Selection_PreR_OnOff_l1.vi"() -> ("output_Selection_PreR_OnOff"=w247:i32)  [unwired: 11 in]
          n138 = call "BRig_dataLC_Selection_PreR_Block_l1.vi"() -> ("output_Selection_PreR_Block"=w246:i32)  [unwired: 11 in]
          n139 = call "BRig_dataLC_Selection_PreR_Prob_l1.vi"() -> ("output_Selection_PreR_Prob"=w245:i32)  [unwired: 11 in]
          n140 = call "BRig_dataLC_Selection_PreR_Delay_l1.vi"() -> ("output_Selection_PreR_Delay"=w244:i32)  [unwired: 11 in]
          n141 = call "BRig_dataLC_Selection_PreR_Count_l1.vi"() -> ("output_Selection_PreR_Count"=w243:i32)  [unwired: 11 in]
          n142 = call "BRig_dataLC_Selection_First_OnOff_l1.vi"() -> ("output_Selection_First_OnOff"=w257:i32)  [unwired: 11 in]
          n143 = call "BRig_dataLC_Selection_First_Block_l1.vi"() -> ("output_Selection_First_Block"=w256:i32)  [unwired: 11 in]
          n144 = call "BRig_dataLC_Selection_First_Prob_l1.vi"() -> ("output_Selection_First_Prob"=w255:i32)  [unwired: 11 in]
          n145 = call "BRig_dataLC_Selection_First_Delay_l1.vi"() -> ("output_Selection_First_Delay"=w254:i32)  [unwired: 11 in]
          n146 = call "BRig_dataLC_Selection_First_Count_l1.vi"() -> ("output_Selection_First_Count"=w253:i32)  [unwired: 11 in]
          n147 = Boolean To (0,1)(Boolean="LC_Sel_First_OnOff") -> (0, 1=w260:i16)
          n148 = Boolean To (0,1)(Boolean="LC_Sel_PreR_OnOff") -> (0, 1=w259:i16)
          n149 = Boolean To (0,1)(Boolean="LC_Sel_PostR_OnOff") -> (0, 1=w258:i16)
          n150 = To Unsigned Word Integer(number=w260) -> (unsigned 16bit integer=w252:u16)
          n151 = To Unsigned Word Integer(number=w259) -> (unsigned 16bit integer=w242:u16)
          n152 = To Unsigned Word Integer(number=w258) -> (unsigned 16bit integer=w232:u16)
          n153 = Replace Array Subset(array=w265, new element #1=w226, index #1=w227, new element #2=w252, index #2=w257, new element #3="LC_Sel_First_Block", index #3=w256, new element #4="LC_Sel_First_Probability", index #4=w255, new element #5="LC_Sel_First_Tdelay", index #5=w254, new element #6="LC_Sel_First_Count", index #6=w253, new element #7=w242, index #7=w247, new element #8="LC_Sel_PreR_Block", index #8=w246, new element #9="LC_Sel_PreR_Probability", index #9=w245, new element #10="LC_Sel_PreR_Tdelay", index #10=w244, new element #11="LC_Sel_PreR_Count", index #11=w243, new element #12=w232, index #12=w237, new element #13="LC_Sel_PostR_Block", index #13=w236, new element #14="LC_Sel_PostR_Probability", index #14=w235, new element #15="LC_Sel_PostR_Tdelay", index #15=w234, new element #16="LC_Sel_PostR_Count", index #16=w233) -> (w264:u16[])
        }
        frame 4 {
          n154 = call "BRig_dataLC_Reward_OnOff_l1.vi"() -> ("output_Reward_OnOff"=w292:i32)  [unwired: 11 in]
          n155 = call "BRig_dataLC_Reward_Block_l1.vi"() -> ("output_Reward_Block"=w291:i32)  [unwired: 11 in]
          n156 = call "BRig_dataLC_Reward_Trial_l1.vi"() -> ("output_Reward_Trial"=w290:i32)  [unwired: 11 in]
          n157 = call "BRig_dataLC_Reward_Prob_l1.vi"() -> ("output_Reward_Prob"=w289:i32)  [unwired: 11 in]
          n158 = call "BRig_dataLC_Reward_Delay_l1.vi"() -> ("output_Reward_Delay"=w288:i32)  [unwired: 11 in]
          n159 = call "BRig_dataLC_Wrong_OnOff_l1.vi"() -> ("output_Wrong_OnOff"=w278:i32)  [unwired: 11 in]
          n160 = call "BRig_dataLC_Wrong_Block_l1.vi"() -> ("output_Wrong_Block"=w277:i32)  [unwired: 11 in]
          n161 = call "BRig_dataLC_Wrong_Trial_l1.vi"() -> ("output_Wrong_Trial"=w276:i32)  [unwired: 11 in]
          n162 = call "BRig_dataLC_Wrong_Prob_l1.vi"() -> ("output_Wrong_Prob"=w275:i32)  [unwired: 11 in]
          n163 = call "BRig_dataLC_Wrong_Delay_l1.vi"() -> ("output_Wrong_Delay"=w274:i32)  [unwired: 11 in]
          n164 = Boolean To (0,1)(Boolean="LC_Reward_OnOff") -> (0, 1=w285:i16)
          n165 = Boolean To (0,1)(Boolean="LC_Wrong_OnOff") -> (0, 1=w284:i16)
          n166 = To Unsigned Word Integer(number=w285) -> (unsigned 16bit integer=w283:u16)
          n167 = To Unsigned Word Integer(number=w284) -> (unsigned 16bit integer=w273:u16)
          n168 = Replace Array Subset(array=w294, new element #1=w267, index #1=w268, new element #2=w283, index #2=w292, new element #3="LC_Reward_Block", index #3=w291, new element #4="LC_Reward_Trial", index #4=w290, new element #5="LC_Reward_Probability", index #5=w289, new element #6="LC_Reward_Tdelay", index #6=w288, new element #7=w273, index #7=w278, new element #8="LC_Wrong_Block", index #8=w277, new element #9="LC_Wrong_Trial", index #9=w276, new element #10="LC_Wrong_Probability", index #10=w275, new element #11="LC_Wrong_Tdelay", index #11=w274) -> (w293:u16[])
        }
        frame 5 {
          w318 = 100.0 ("y")
          n169 = call "BRig_dataExp_LED_baseline_l1.vi"() -> ("output_LED_baseline_l1"=w295:i32)  [unwired: 11 in]
          n170 = call "BRig_dataExp_L_freq_l1.vi"() -> ("output_L_freq_l1"=w317:i32)  [unwired: 11 in]
          n171 = call "BRig_dataExp_L_T_l1.vi"() -> ("output_L_T_l1"=w316:i32)  [unwired: 11 in]
          n172 = call "BRig_dataExp_L_Tpeak_l1.vi"() -> ("output_L_Tpeak_l1"=w315:i32)  [unwired: 11 in]
          n173 = call "BRig_dataExp_L_Tshutter_l1.vi"() -> ("output_L_Tshutter_l1"=w314:i32)  [unwired: 11 in]
          n174 = call "BRig_dataExp_L_power_min_l1.vi"() -> ("output_L_power_min_l1"=w313:i32)  [unwired: 11 in]
          n175 = call "BRig_dataExp_L_power_max_l1.vi"() -> ("output_L_power_max_l1"=w312:i32)  [unwired: 11 in]
          n176 = call "BRig_dataExp_L_power_step_l1.vi"() -> ("output_L_power_step_l1"=w311:i32)  [unwired: 11 in]
          n177 = call "BRig_dataExp_L_Ttotal_l1.vi"() -> ("output_L_Ttotal_l1"=w305:i32)  [unwired: 11 in]
          n178 = Boolean To (0,1)(Boolean="LED_baseline") -> (0, 1=w330:i16)
          n179 = To Unsigned Word Integer(number=w330) -> (unsigned 16bit integer=w328:u16)
          n180 = Multiply(x="Laser_power_min", y=w318) -> (x*y=w322:dbl)
          n181 = Multiply(x="Laser_power_max", y=w318) -> (x*y=w324:dbl)
          n182 = Multiply(x="Laser_power_step", y=w318) -> (x*y=w327:dbl)
          n183 = Round To Nearest(number=w322) -> (nearest integer value=w321:dbl)
          n184 = Round To Nearest(number=w324) -> (nearest integer value=w323:dbl)
          n185 = Round To Nearest(number=w327) -> (nearest integer value=w326:dbl)
          n186 = To Unsigned Word Integer(number=w321) -> (unsigned 16bit integer=w308:u16)
          n187 = To Unsigned Word Integer(number=w323) -> (unsigned 16bit integer=w309:u16)
          n188 = To Unsigned Word Integer(number=w326) -> (unsigned 16bit integer=w310:u16)
          n189 = Add(x="Laser_T", y="Laser_Tshutter") -> (x+y=w302:u16)
          n190 = Replace Array Subset(array=w299, new element=w296, index=w297) -> (w298:u16[])
          n191 = Replace Array Subset(array=w301, new element #1=w328, index #1=w295, new element #2="Laser_Freq", index #2=w317, new element #3="Laser_T", index #3=w316, new element #4="Laser_Tpeak", index #4=w315, new element #5="Laser_Tshutter", index #5=w314, new element #6=w308, index #6=w313, new element #7=w309, index #7=w312, new element #8=w310, index #8=w311, new element #9=w302, index #9=w305) -> (w300:u16[])
        }
        frame 6 {
          n192 = call "BRig_dataExp_L_freq_l1.vi"() -> ("output_L_freq_l1"=w333:i32)  [unwired: 11 in]
          n193 = call "BRig_dataExp_L_T_l1.vi"() -> ("output_L_T_l1"=w334:i32)  [unwired: 11 in]
          n194 = call "BRig_dataExp_L_Tpeak_l1.vi"() -> ("output_L_Tpeak_l1"=w332:i32)  [unwired: 11 in]
          n195 = call "BRig_dataExp_L_Tshutter_l1.vi"() -> ("output_L_Tshutter_l1"=w331:i32)  [unwired: 11 in]
          n196 = Replace Array Subset(array=w338, new element=w335, index=w336) -> (w337:u16[])
          n197 = call "BRig_RT__Case_Idle__calc_LaserPulse.vi"("input_dataExp_L_Tshutter"=w331, "input_dataExp_L_Tpeak"=w332, "input_dataExp_L_T"=w334, "input_dataExp_L_freq"=w333, "input_dataExp"=w340) -> ("output_cluster"=→"LaserPulseTrain":cluster{u16[], u16[]})  [unwired: 6 in]
        }
      }
    }
    frame True {
      w440 = 100.0 ("y")
      n198 = call "BRig_dataLC_ENL_First_OnOff_l1.vi"() -> ("output_ENL_First_OnOff"=w583:i32)  [unwired: 11 in]
      n199 = call "BRig_dataLC_ENL_First_Block_l1.vi"() -> ("output_ENL_First_Block"=w582:i32)  [unwired: 11 in]
      n200 = call "BRig_dataLC_ENL_First_Prob_l1.vi"() -> ("output_ENL_First_Prob"=w581:i32)  [unwired: 11 in]
      n201 = call "BRig_dataLC_ENL_First_Delay_l1.vi"() -> ("output_ENL_First_Delay"=w580:i32)  [unwired: 11 in]
      n202 = call "BRig_dataLC_ENL_First_DelayOpt_l1.vi"() -> ("output_ENL_First_DelayOpt"=w579:i32)  [unwired: 11 in]
      n203 = call "BRig_dataLC_ENL_First_Count_l1.vi"() -> ("output_ENL_First_Count"=w578:i32)  [unwired: 11 in]
      n204 = call "BRig_dataLC_ENL_PreR_OnOff_l1.vi"() -> ("output_ENL_PreR_OnOff"=w577:i32)  [unwired: 11 in]
      n205 = call "BRig_dataLC_ENL_PreR_Block_l1.vi"() -> ("output_ENL_PreR_Block"=w576:i32)  [unwired: 11 in]
      n206 = call "BRig_dataLC_ENL_PreR_Prob_l1.vi"() -> ("output_ENL_PreR_Prob"=w575:i32)  [unwired: 11 in]
      n207 = call "BRig_dataLC_ENL_PreR_Delay_l1.vi"() -> ("output_ENL_PreR_Delay"=w574:i32)  [unwired: 11 in]
      n208 = call "BRig_dataLC_ENL_PreR_DelayOpt_l1.vi"() -> ("output_ENL_PreR_DelayOpt"=w573:i32)  [unwired: 11 in]
      n209 = call "BRig_dataLC_ENL_PreR_Count_l1.vi"() -> ("output_ENL_PreR_Count"=w572:i32)  [unwired: 11 in]
      n210 = call "BRig_dataLC_ENL_PostR_OnOff_l1.vi"() -> ("output_ENL_PostR_OnOff"=w571:i32)  [unwired: 11 in]
      n211 = call "BRig_dataLC_ENL_PostR_Block_l1.vi"() -> ("output_ENL_PostR_Block"=w570:i32)  [unwired: 11 in]
      n212 = call "BRig_dataLC_ENL_PostR_Prob_l1.vi"() -> ("output_ENL_PostR_Prob"=w569:i32)  [unwired: 11 in]
      n213 = call "BRig_dataLC_ENL_PostR_Delay_l1.vi"() -> ("output_ENL_PostR_Delay"=w568:i32)  [unwired: 11 in]
      n214 = call "BRig_dataLC_ENL_PostR_DelayOpt_l1.vi"() -> ("output_ENL_PostR_DelayOpt"=w567:i32)  [unwired: 11 in]
      n215 = call "BRig_dataLC_ENL_PostR_Count_l1.vi"() -> ("output_ENL_PostR_Count"=w566:i32)  [unwired: 11 in]
      n216 = call "BRig_dataLC_ENL2_First_OnOff_l1.vi"() -> ("output_ENL2_First_OnOff"=w425:i32)  [unwired: 11 in]
      n217 = call "BRig_dataLC_ENL2_First_Block_l1.vi"() -> ("output_ENL2_First_Block"=w424:i32)  [unwired: 11 in]
      n218 = call "BRig_dataLC_ENL2_First_Prob_l1.vi"() -> ("output_ENL2_First_Prob"=w423:i32)  [unwired: 11 in]
      n219 = call "BRig_dataLC_ENL2_First_Delay_l1.vi"() -> ("output_ENL2_First_Delay"=w422:i32)  [unwired: 11 in]
      n220 = call "BRig_dataLC_ENL2_First_DelayOpt_l1.vi"() -> ("output_ENL2_First_DelayOpt"=w421:i32)  [unwired: 11 in]
      n221 = call "BRig_dataLC_ENL2_First_Count_l1.vi"() -> ("output_ENL2_First_Count"=w420:i32)  [unwired: 11 in]
      n222 = call "BRig_dataLC_ENL2_PreR_OnOff_l1.vi"() -> ("output_ENL2_PreR_OnOff"=w419:i32)  [unwired: 11 in]
      n223 = call "BRig_dataLC_ENL2_PreR_Block_l1.vi"() -> ("output_ENL2_PreR_Block"=w418:i32)  [unwired: 11 in]
      n224 = call "BRig_dataLC_ENL2_PreR_Prob_l1.vi"() -> ("output_ENL2_PreR_Prob"=w417:i32)  [unwired: 11 in]
      n225 = call "BRig_dataLC_ENL2_PreR_Delay_l1.vi"() -> ("output_ENL2_PreR_Delay"=w416:i32)  [unwired: 11 in]
      n226 = call "BRig_dataLC_ENL2_PreR_DelayOpt_l1.vi"() -> ("output_ENL2_PreR_DelayOpt"=w415:i32)  [unwired: 11 in]
      n227 = call "BRig_dataLC_ENL2_PreR_Count_l1.vi"() -> ("output_ENL2_PreR_Count"=w414:i32)  [unwired: 11 in]
      n228 = call "BRig_dataLC_ENL2_PostR_OnOff_l1.vi"() -> ("output_ENL2_PostR_OnOff"=w413:i32)  [unwired: 11 in]
      n229 = call "BRig_dataLC_ENL2_PostR_Block_l1.vi"() -> ("output_ENL2_PostR_Block"=w412:i32)  [unwired: 11 in]
      n230 = call "BRig_dataLC_ENL2_PostR_Prob_l1.vi"() -> ("output_ENL2_PostR_Prob"=w411:i32)  [unwired: 11 in]
      n231 = call "BRig_dataLC_ENL2_PostR_Delay_l1.vi"() -> ("output_ENL2_PostR_Delay"=w410:i32)  [unwired: 11 in]
      n232 = call "BRig_dataLC_ENL2_PostR_DelayOpt_l1.vi"() -> ("output_ENL2_PostR_DelayOpt"=w409:i32)  [unwired: 11 in]
      n233 = call "BRig_dataLC_ENL2_PostR_Count_l1.vi"() -> ("output_ENL2_PostR_Count"=w408:i32)  [unwired: 11 in]
      n234 = Index Array(array=w462, index #1=w583, index #2=w582, index #3=w581, index #4=w580, index #5=w579, index #6=w578, index #7=w577, index #8=w576, index #9=w575, index #10=w574, index #11=w573, index #12=w572, index #13=w571, index #14=w570, index #15=w569, index #16=w568, index #17=w567, index #18=w566) -> (element #1=w559:u16, element #2=w558:u16, element #3=w557:u16, element #4=w556:u16, element #5=w555:u16, element #6=w554:u16, element #7=w553:u16, element #8=w552:u16, element #9=w551:u16, element #10=w550:u16, element #11=w549:u16, element #12=w548:u16, element #13=w547:u16, element #14=w546:u16, element #15=w545:u16, element #16=w544:u16, element #17=w543:u16, element #18=w542:u16)
      n235 = Index Array(array=w377, index #1=w425, index #2=w424, index #3=w423, index #4=w422, index #5=w421, index #6=w420, index #7=w419, index #8=w418, index #9=w417, index #10=w416, index #11=w415, index #12=w414, index #13=w413, index #14=w412, index #15=w411, index #16=w410, index #17=w409, index #18=w408) -> (element #1=w384:u16, element #2=w385:u16, element #3=w386:u16, element #4=w387:u16, element #5=w388:u16, element #6=w389:u16, element #7=w390:u16, element #8=w391:u16, element #9=w392:u16, element #10=w393:u16, element #11=w394:u16, element #12=w395:u16, element #13=w397:u16, element #14=w398:u16, element #15=w399:u16, element #16=w400:u16, element #17=w401:u16, element #18=w402:u16)
      n236 = Not Equal To 0?(x=w559) -> (x != 0?=w565:bool)
      n237 = Not Equal To 0?(x=w555) -> (x != 0?=w564:bool)
      n238 = Not Equal To 0?(x=w553) -> (x != 0?=w563:bool)
      n239 = Not Equal To 0?(x=w549) -> (x != 0?=w562:bool)
      n240 = Not Equal To 0?(x=w547) -> (x != 0?=w561:bool)
      n241 = Not Equal To 0?(x=w543) -> (x != 0?=w560:bool)
      n242 = local write "LC_ENL_First_OnOff"(w565) -> ()
      n243 = local write "LC_ENL_First_Block"(w558) -> ()
      n244 = local write "LC_ENL_First_Probability"(w557) -> ()
      n245 = local write "LC_ENL_First_Tdelay"(w556) -> ()
      n246 = local write "LC_ENL_First_delayOpt"(w564) -> ()
      n247 = local write "LC_ENL_First_Count"(w554) -> ()
      n248 = local write "LC_ENL_PreR_OnOff"(w563) -> ()
      n249 = local write "LC_ENL_PreR_Block"(w552) -> ()
      n250 = local write "LC_ENL_PreR_Probability"(w551) -> ()
      n251 = local write "LC_ENL_PreR_Tdelay"(w550) -> ()
      n252 = local write "LC_ENL_PreR_delayOpt"(w562) -> ()
      n253 = local write "LC_ENL_PreR_Count"(w548) -> ()
      n254 = local write "LC_ENL_PostR_OnOff"(w561) -> ()
      n255 = local write "LC_ENL_PostR_Block"(w546) -> ()
      n256 = local write "LC_ENL_PostR_Probability"(w545) -> ()
      n257 = local write "LC_ENL_PostR_Tdelay"(w544) -> ()
      n258 = local write "LC_ENL_PostR_delayOpt"(w560) -> ()
      n259 = local write "LC_ENL_PostR_Count"(w542) -> ()
      n260 = Not Equal To 0?(x=w384) -> (x != 0?=w405:bool)
      n261 = Not Equal To 0?(x=w388) -> (x != 0?=w406:bool)
      n262 = Not Equal To 0?(x=w390) -> (x != 0?=w404:bool)
      n263 = Not Equal To 0?(x=w394) -> (x != 0?=w407:bool)
      n264 = Not Equal To 0?(x=w397) -> (x != 0?=w403:bool)
      n265 = Not Equal To 0?(x=w401) -> (x != 0?=w396:bool)
      n266 = local write "LC_ENL2_First_OnOff"(w405) -> ()
      n267 = local write "LC_ENL2_First_Block"(w385) -> ()
      n268 = local write "LC_ENL2_First_Probability"(w386) -> ()
      n269 = local write "LC_ENL2_First_Tdelay"(w387) -> ()
      n270 = local write "LC_ENL2_First_delayOpt"(w406) -> ()
      n271 = local write "LC_ENL2_First_Count"(w389) -> ()
      n272 = local write "LC_ENL2_PreR_OnOff"(w404) -> ()
      n273 = local write "LC_ENL2_PreR_Block"(w391) -> ()
      n274 = local write "LC_ENL2_PreR_Probability"(w392) -> ()
      n275 = local write "LC_ENL2_PreR_Tdelay"(w393) -> ()
      n276 = local write "LC_ENL2_PreR_delayOpt"(w407) -> ()
      n277 = local write "LC_ENL2_PreR_Count"(w395) -> ()
      n278 = local write "LC_ENL2_PostR_OnOff"(w403) -> ()
      n279 = local write "LC_ENL2_PostR_Block"(w398) -> ()
      n280 = local write "LC_ENL2_PostR_Probability"(w399) -> ()
      n281 = local write "LC_ENL2_PostR_Tdelay"(w400) -> ()
      n282 = local write "LC_ENL2_PostR_delayOpt"(w396) -> ()
      n283 = local write "LC_ENL2_PostR_Count"(w402) -> ()
      n284 = call "BRig_dataLC_Cue_PreR_OnOff_l1.vi"() -> ("output_Cue_PreR_OnOff"=w430:i32)  [unwired: 11 in]
      n285 = call "BRig_dataLC_Cue_PreR_Block_l1.vi"() -> ("output_Cue_PreR_Block"=w429:i32)  [unwired: 11 in]
      n286 = call "BRig_dataLC_Cue_PreR_Prob_l1.vi"() -> ("output_Cue_PreR_Prob"=w428:i32)  [unwired: 11 in]
      n287 = call "BRig_dataLC_Cue_PreR_Delay_l1.vi"() -> ("output_Cue_PreR_Delay"=w427:i32)  [unwired: 11 in]
      n288 = call "BRig_dataLC_Cue_PreR_DelayOpt_l1.vi"() -> ("output_Cue_PreR_DelayOpt"=w426:i32)  [unwired: 11 in]
      n289 = call "BRig_dataLC_Cue_PreR_Count_l1.vi"() -> ("output_Cue_PreR_Count"=w431:i32)  [unwired: 11 in]
      n290 = call "BRig_dataLC_Cue_First_OnOff_l1.vi"() -> ("output_Cue_First_OnOff"=w589:i32)  [unwired: 11 in]
      n291 = call "BRig_dataLC_Cue_First_Block_l1.vi"() -> ("output_Cue_First_Block"=w588:i32)  [unwired: 11 in]
      n292 = call "BRig_dataLC_Cue_First_Prob_l1.vi"() -> ("output_Cue_First_Prob"=w587:i32)  [unwired: 11 in]
      n293 = call "BRig_dataLC_Cue_First_Delay_l1.vi"() -> ("output_Cue_First_Delay"=w586:i32)  [unwired: 11 in]
      n294 = call "BRig_dataLC_Cue_First_DelayOpt_l1.vi"() -> ("output_Cue_First_DelayOpt"=w585:i32)  [unwired: 11 in]
      n295 = call "BRig_dataLC_Cue_First_Count_l1.vi"() -> ("output_Cue_First_Count"=w584:i32)  [unwired: 11 in]
      n296 = call "BRig_dataLC_Cue_PostR_OnOff_l1.vi"() -> ("output_Cue_PostR_OnOff"=w436:i32)  [unwired: 11 in]
      n297 = call "BRig_dataLC_Cue_PostR_Block_l1.vi"() -> ("output_Cue_PostR_Block"=w435:i32)  [unwired: 11 in]
      n298 = call "BRig_dataLC_Cue_PostR_Prob_l1.vi"() -> ("output_Cue_PostR_Prob"=w434:i32)  [unwired: 11 in]
      n299 = call "BRig_dataLC_Cue_PostR_Delay_l1.vi"() -> ("output_Cue_PostR_Delay"=w433:i32)  [unwired: 11 in]
      n300 = call "BRig_dataLC_Cue_PostR_DelayOpt_l1.vi"() -> ("output_Cue_PostR_DelayOpt"=w432:i32)  [unwired: 11 in]
      n301 = call "BRig_dataLC_Cue_PostR_Count_l1.vi"() -> ("output_Cue_PostR_Count"=w437:i32)  [unwired: 11 in]
      n302 = call "BRig_dataExp_LED_baseline_Cue.vi"() -> ("output_LED_baseline_Cue"=w461:i32)  [unwired: 11 in]
      n303 = call "BRig_dataExp_L_freq_l1.vi"() -> ("output_L_freq_l1"=w460:i32)  [unwired: 11 in]
      n304 = call "BRig_dataExp_L_T_l1.vi"() -> ("output_L_T_l1"=w459:i32)  [unwired: 11 in]
      n305 = call "BRig_dataExp_L_Tpeak_l1.vi"() -> ("output_L_Tpeak_l1"=w458:i32)  [unwired: 11 in]
      n306 = call "BRig_dataExp_L_Tshutter_l1.vi"() -> ("output_L_Tshutter_l1"=w457:i32)  [unwired: 11 in]
      n307 = call "BRig_dataExp_L_power_min_l1.vi"() -> ("output_L_power_min_l1"=w456:i32)  [unwired: 11 in]
      n308 = call "BRig_dataExp_L_power_max_l1.vi"() -> ("output_L_power_max_l1"=w455:i32)  [unwired: 11 in]
      n309 = call "BRig_dataExp_L_power_step_l1.vi"() -> ("output_L_power_step_l1"=w454:i32)  [unwired: 11 in]
      n310 = Index Array(array=w462, index #1=w589, index #2=w588, index #3=w587, index #4=w586, index #5=w585, index #6=w584, index #7=w430, index #8=w429, index #9=w428, index #10=w427, index #11=w426, index #12=w431, index #13=w436, index #14=w435, index #15=w434, index #16=w433, index #17=w432, index #18=w437) -> (element #1=w535:u16, element #2=w534:u16, element #3=w533:u16, element #4=w532:u16, element #5=w531:u16, element #6=w530:u16, element #7=w529:u16, element #8=w528:u16, element #9=w527:u16, element #10=w526:u16, element #11=w525:u16, element #12=w524:u16, element #13=w523:u16, element #14=w522:u16, element #15=w521:u16, element #16=w520:u16, element #17=w519:u16, element #18=w518:u16)
      n311 = Index Array(array=w377, index #1=w461, index #2=w460, index #3=w459, index #4=w458, index #5=w457, index #6=w456, index #7=w455, index #8=w454) -> (element #1=w453:u16, element #2=w451:u16, element #3=w450:u16, element #4=w449:u16, element #5=w448:u16, element #6=w447:u16, element #7=w446:u16, element #8=w445:u16)
      n312 = To Double Precision Float(number=w447) -> (double precision float=w444:dbl)
      n313 = To Double Precision Float(number=w446) -> (double precision float=w439:dbl)
      n314 = To Double Precision Float(number=w445) -> (double precision float=w438:dbl)
      n315 = Not Equal To 0?(x=w535) -> (x != 0?=w541:bool)
      n316 = Not Equal To 0?(x=w531) -> (x != 0?=w540:bool)
      n317 = Not Equal To 0?(x=w529) -> (x != 0?=w539:bool)
      n318 = Not Equal To 0?(x=w525) -> (x != 0?=w538:bool)
      n319 = Not Equal To 0?(x=w523) -> (x != 0?=w537:bool)
      n320 = Not Equal To 0?(x=w519) -> (x != 0?=w536:bool)
      n321 = Divide(x=w444, y=w440) -> (x/y=w443:dbl)
      n322 = Divide(x=w439, y=w440) -> (x/y=w442:dbl)
      n323 = Divide(x=w438, y=w440) -> (x/y=w441:dbl)
      n324 = local write "LC_Cue_First_OnOff"(w541) -> ()
      n325 = local write "LC_Cue_First_Block"(w534) -> ()
      n326 = local write "LC_Cue_First_Probability"(w533) -> ()
      n327 = local write "LC_Cue_First_Tdelay"(w532) -> ()
      n328 = local write "LC_Cue_First_delayOpt"(w540) -> ()
      n329 = local write "LC_Cue_First_Count"(w530) -> ()
      n330 = local write "LC_Cue_PreR_OnOff"(w539) -> ()
      n331 = local write "LC_Cue_PreR_Block"(w528) -> ()
      n332 = local write "LC_Cue_PreR_Probability"(w527) -> ()
      n333 = local write "LC_Cue_PreR_Tdelay"(w526) -> ()
      n334 = local write "LC_Cue_PreR_delayOpt"(w538) -> ()
      n335 = local write "LC_Cue_PreR_Count"(w524) -> ()
      n336 = local write "LC_Cue_PostR_OnOff"(w537) -> ()
      n337 = local write "LC_Cue_PostR_Block"(w522) -> ()
      n338 = local write "LC_Cue_PostR_Probability"(w521) -> ()
      n339 = local write "LC_Cue_PostR_Tdelay"(w520) -> ()
      n340 = local write "LC_Cue_PostR_delayOpt"(w536) -> ()
      n341 = local write "LC_Cue_PostR_Count"(w518) -> ()
      n342 = Not Equal To 0?(x=w453) -> (x != 0?=w452:bool)
      n343 = call "BRig_dataLC_Cue2_First_OnOff_l1.vi"() -> ("output_Cue2_First_OnOff"=w359:i32)  [unwired: 11 in]
      n344 = call "BRig_dataLC_Cue2_First_Block_l1.vi"() -> ("output_Cue2_First_Block"=w360:i32)  [unwired: 11 in]
      n345 = call "BRig_dataLC_Cue2_First_Prob_l1.vi"() -> ("output_Cue2_First_Prob"=w361:i32)  [unwired: 11 in]
      n346 = call "BRig_dataLC_Cue2_First_Delay_l1.vi"() -> ("output_Cue2_First_Delay"=w362:i32)  [unwired: 11 in]
      n347 = call "BRig_dataLC_Cue2_First_DelayOpt_l1.vi"() -> ("output_Cue2_First_DelayOpt"=w363:i32)  [unwired: 11 in]
      n348 = call "BRig_dataLC_Cue2_First_Count_l1.vi"() -> ("output_Cue2_First_Count"=w364:i32)  [unwired: 11 in]
      n349 = call "BRig_dataLC_Cue2_PreR_OnOff_l1.vi"() -> ("output_Cue2_PreR_OnOff"=w365:i32)  [unwired: 11 in]
      n350 = call "BRig_dataLC_Cue2_PreR_Block_l1.vi"() -> ("output_Cue2_PreR_Block"=w366:i32)  [unwired: 11 in]
      n351 = call "BRig_dataLC_Cue2_PreR_Prob_l1.vi"() -> ("output_Cue2_PreR_Prob"=w367:i32)  [unwired: 11 in]
      n352 = call "BRig_dataLC_Cue2_PreR_Delay_l1.vi"() -> ("output_Cue2_PreR_Delay"=w368:i32)  [unwired: 11 in]
      n353 = call "BRig_dataLC_Cue2_PreR_DelayOpt_l1.vi"() -> ("output_Cue2_PreR_DelayOpt"=w369:i32)  [unwired: 11 in]
      n354 = call "BRig_dataLC_Cue2_PreR_Count_l1.vi"() -> ("output_Cue2_PreR_Count"=w370:i32)  [unwired: 11 in]
      n355 = call "BRig_dataLC_Cue2_PostR_OnOff_l1.vi"() -> ("output_Cue2_PostR_OnOff"=w371:i32)  [unwired: 11 in]
      n356 = call "BRig_dataLC_Cue2_PostR_Block_l1.vi"() -> ("output_Cue2_PostR_Block"=w372:i32)  [unwired: 11 in]
      n357 = call "BRig_dataLC_Cue2_PostR_Prob_l1.vi"() -> ("output_Cue2_PostR_Prob"=w373:i32)  [unwired: 11 in]
      n358 = call "BRig_dataLC_Cue2_PostR_Delay_l1.vi"() -> ("output_Cue2_PostR_Delay"=w374:i32)  [unwired: 11 in]
      n359 = call "BRig_dataLC_Cue2_PostR_DelayOpt_l1.vi"() -> ("output_Cue2_PostR_DelayOpt"=w375:i32)  [unwired: 11 in]
      n360 = call "BRig_dataLC_Cue2_PostR_Count_l1.vi"() -> ("output_Cue2_PostR_Count"=w376:i32)  [unwired: 11 in]
      n361 = local write "LED_baseline"(w452) -> ()
      n362 = local write "Laser_Freq"(w451) -> ()
      n363 = local write "Laser_T"(w450) -> ()
      n364 = local write "Laser_Tpeak"(w449) -> ()
      n365 = local write "Laser_Tshutter"(w448) -> ()
      n366 = local write "Laser_power_min"(w443) -> ()
      n367 = local write "Laser_power_max"(w442) -> ()
      n368 = local write "Laser_power_step"(w441) -> ()
      n369 = Index Array(array=w377, index #1=w359, index #2=w360, index #3=w361, index #4=w362, index #5=w363, index #6=w364, index #7=w365, index #8=w366, index #9=w367, index #10=w368, index #11=w369, index #12=w370, index #13=w371, index #14=w372, index #15=w373, index #16=w374, index #17=w375, index #18=w376) -> (element #1=w378:u16, element #2=w355:u16, element #3=w354:u16, element #4=w353:u16, element #5=w379:u16, element #6=w356:u16, element #7=w380:u16, element #8=w350:u16, element #9=w349:u16, element #10=w348:u16, element #11=w381:u16, element #12=w347:u16, element #13=w382:u16, element #14=w344:u16, element #15=w343:u16, element #16=w342:u16, element #17=w383:u16, element #18=w341:u16)
      n370 = call "BRig_dataLC_Selection_PostR_OnOff_l1.vi"() -> ("output_Selection_PostR_OnOff"=w507:i32)  [unwired: 11 in]
      n371 = call "BRig_dataLC_Selection_PostR_Block_l1.vi"() -> ("output_Selection_PostR_Block"=w506:i32)  [unwired: 11 in]
      n372 = call "BRig_dataLC_Selection_PostR_Prob_l1.vi"() -> ("output_Selection_PostR_Prob"=w505:i32)  [unwired: 11 in]
      n373 = call "BRig_dataLC_Selection_PostR_Delay_l1.vi"() -> ("output_Selection_PostR_Delay"=w504:i32)  [unwired: 11 in]
      n374 = call "BRig_dataLC_Selection_PostR_Count_l1.vi"() -> ("output_Selection_PostR_Count"=w503:i32)  [unwired: 11 in]
      n375 = call "BRig_dataLC_Selection_PreR_OnOff_l1.vi"() -> ("output_Selection_PreR_OnOff"=w512:i32)  [unwired: 11 in]
      n376 = call "BRig_dataLC_Selection_PreR_Block_l1.vi"() -> ("output_Selection_PreR_Block"=w511:i32)  [unwired: 11 in]
      n377 = call "BRig_dataLC_Selection_PreR_Prob_l1.vi"() -> ("output_Selection_PreR_Prob"=w510:i32)  [unwired: 11 in]
      n378 = call "BRig_dataLC_Selection_PreR_Delay_l1.vi"() -> ("output_Selection_PreR_Delay"=w509:i32)  [unwired: 11 in]
      n379 = call "BRig_dataLC_Selection_PreR_Count_l1.vi"() -> ("output_Selection_PreR_Count"=w508:i32)  [unwired: 11 in]
      n380 = call "BRig_dataLC_Selection_First_OnOff_l1.vi"() -> ("output_Selection_First_OnOff"=w517:i32)  [unwired: 11 in]
      n381 = call "BRig_dataLC_Selection_First_Block_l1.vi"() -> ("output_Selection_First_Block"=w516:i32)  [unwired: 11 in]
      n382 = call "BRig_dataLC_Selection_First_Prob_l1.vi"() -> ("output_Selection_First_Prob"=w515:i32)  [unwired: 11 in]
      n383 = call "BRig_dataLC_Selection_First_Delay_l1.vi"() -> ("output_Selection_First_Delay"=w514:i32)  [unwired: 11 in]
      n384 = call "BRig_dataLC_Selection_First_Count_l1.vi"() -> ("output_Selection_First_Count"=w513:i32)  [unwired: 11 in]
      n385 = call "BRig_dataLC_Reward_OnOff_l1.vi"() -> ("output_Reward_OnOff"=w484:i32)  [unwired: 11 in]
      n386 = call "BRig_dataLC_Reward_Block_l1.vi"() -> ("output_Reward_Block"=w483:i32)  [unwired: 11 in]
      n387 = call "BRig_dataLC_Reward_Trial_l1.vi"() -> ("output_Reward_Trial"=w482:i32)  [unwired: 11 in]
      n388 = call "BRig_dataLC_Reward_Prob_l1.vi"() -> ("output_Reward_Prob"=w481:i32)  [unwired: 11 in]
      n389 = call "BRig_dataLC_Reward_Delay_l1.vi"() -> ("output_Reward_Delay"=w480:i32)  [unwired: 11 in]
      n390 = call "BRig_dataLC_Wrong_OnOff_l1.vi"() -> ("output_Wrong_OnOff"=w479:i32)  [unwired: 11 in]
      n391 = call "BRig_dataLC_Wrong_Block_l1.vi"() -> ("output_Wrong_Block"=w478:i32)  [unwired: 11 in]
      n392 = call "BRig_dataLC_Wrong_Trial_l1.vi"() -> ("output_Wrong_Trial"=w477:i32)  [unwired: 11 in]
      n393 = call "BRig_dataLC_Wrong_Prob_l1.vi"() -> ("output_Wrong_Prob"=w476:i32)  [unwired: 11 in]
      n394 = call "BRig_dataLC_Wrong_Delay_l1.vi"() -> ("output_Wrong_Delay"=w475:i32)  [unwired: 11 in]
      n395 = Not Equal To 0?(x=w378) -> (x != 0?=w358:bool)
      n396 = Not Equal To 0?(x=w379) -> (x != 0?=w357:bool)
      n397 = Not Equal To 0?(x=w380) -> (x != 0?=w351:bool)
      n398 = Not Equal To 0?(x=w381) -> (x != 0?=w352:bool)
      n399 = Not Equal To 0?(x=w382) -> (x != 0?=w346:bool)
      n400 = Not Equal To 0?(x=w383) -> (x != 0?=w345:bool)
      n401 = Index Array(array=w462, index #1=w484, index #2=w483, index #3=w482, index #4=w481, index #5=w480, index #6=w479, index #7=w478, index #8=w477, index #9=w476, index #10=w475) -> (element #1=w472:u16, element #2=w471:u16, element #3=w470:u16, element #4=w469:u16, element #5=w468:u16, element #6=w467:u16, element #7=w466:u16, element #8=w465:u16, element #9=w464:u16, element #10=w463:u16)
      n402 = local write "LC_Cue2_First_OnOff"(w358) -> ()
      n403 = local write "LC_Cue2_First_Block"(w355) -> ()
      n404 = local write "LC_Cue2_First_Probability"(w354) -> ()
      n405 = local write "LC_Cue2_First_Tdelay"(w353) -> ()
      n406 = local write "LC_Cue2_First_delayOpt"(w357) -> ()
      n407 = local write "LC_Cue2_First_Count"(w356) -> ()
      n408 = local write "LC_Cue2_PreR_OnOff"(w351) -> ()
      n409 = local write "LC_Cue2_PreR_Block"(w350) -> ()
      n410 = local write "LC_Cue2_PreR_Probability"(w349) -> ()
      n411 = local write "LC_Cue2_PreR_Tdelay"(w348) -> ()
      n412 = local write "LC_Cue2_PreR_delayOpt"(w352) -> ()
      n413 = local write "LC_Cue2_PreR_Count"(w347) -> ()
      n414 = local write "LC_Cue2_PostR_OnOff"(w346) -> ()
      n415 = local write "LC_Cue2_PostR_Block"(w344) -> ()
      n416 = local write "LC_Cue2_PostR_Probability"(w343) -> ()
      n417 = local write "LC_Cue2_PostR_Tdelay"(w342) -> ()
      n418 = local write "LC_Cue2_PostR_delayOpt"(w345) -> ()
      n419 = local write "LC_Cue2_PostR_Count"(w341) -> ()
      n420 = Index Array(array=w462, index #1=w517, index #2=w516, index #3=w515, index #4=w514, index #5=w513, index #6=w512, index #7=w511, index #8=w510, index #9=w509, index #10=w508, index #11=w507, index #12=w506, index #13=w505, index #14=w504, index #15=w503) -> (element #1=w499:u16, element #2=w498:u16, element #3=w497:u16, element #4=w496:u16, element #5=w495:u16, element #6=w494:u16, element #7=w493:u16, element #8=w492:u16, element #9=w491:u16, element #10=w490:u16, element #11=w489:u16, element #12=w488:u16, element #13=w487:u16, element #14=w486:u16, element #15=w485:u16)
      n421 = Not Equal To 0?(x=w472) -> (x != 0?=w474:bool)
      n422 = Not Equal To 0?(x=w467) -> (x != 0?=w473:bool)
      n423 = Not Equal To 0?(x=w499) -> (x != 0?=w502:bool)
      n424 = Not Equal To 0?(x=w494) -> (x != 0?=w501:bool)
      n425 = Not Equal To 0?(x=w489) -> (x != 0?=w500:bool)
      n426 = local write "LC_Reward_OnOff"(w474) -> ()
      n427 = local write "LC_Reward_Block"(w471) -> ()
      n428 = local write "LC_Reward_Trial"(w470) -> ()
      n429 = local write "LC_Reward_Probability"(w469) -> ()
      n430 = local write "LC_Reward_Tdelay"(w468) -> ()
      n431 = local write "LC_Wrong_OnOff"(w473) -> ()
      n432 = local write "LC_Wrong_Block"(w466) -> ()
      n433 = local write "LC_Wrong_Trial"(w465) -> ()
      n434 = local write "LC_Wrong_Probability"(w464) -> ()
      n435 = local write "LC_Wrong_Tdelay"(w463) -> ()
      n436 = local write "LC_Sel_First_OnOff"(w502) -> ()
      n437 = local write "LC_Sel_First_Block"(w498) -> ()
      n438 = local write "LC_Sel_First_Probability"(w497) -> ()
      n439 = local write "LC_Sel_First_Tdelay"(w496) -> ()
      n440 = local write "LC_Sel_First_Count"(w495) -> ()
      n441 = local write "LC_Sel_PreR_OnOff"(w501) -> ()
      n442 = local write "LC_Sel_PreR_Block"(w493) -> ()
      n443 = local write "LC_Sel_PreR_Probability"(w492) -> ()
      n444 = local write "LC_Sel_PreR_Tdelay"(w491) -> ()
      n445 = local write "LC_Sel_PreR_Count"(w490) -> ()
      n446 = local write "LC_Sel_PostR_OnOff"(w500) -> ()
      n447 = local write "LC_Sel_PostR_Block"(w488) -> ()
      n448 = local write "LC_Sel_PostR_Probability"(w487) -> ()
      n449 = local write "LC_Sel_PostR_Tdelay"(w486) -> ()
      n450 = local write "LC_Sel_PostR_Count"(w485) -> ()
    }
  }
  "output_dataLC" <- w4
  "output_dataExp" <- w1
